vi "SDK Sample.vi"() -> ()   [LabVIEW 2015]
uses:
  sub/Mode.ctl
  sub/global.vi
panel:
  out "Depth":i8
  out "nDeviceNoList":u32[](array[numeric])
  out "MaxSize":cluster{"pWidth":u32, "pHeight":u32}={"pWidth"=2048, "pHeight"=2048}
  out "pDetectNumInfoLV":T1
  out "SetupCover2":string
  out "SetupCover1":string
  out "FLG_LiveStop":u16(ring) items=["Live", "Get", "Stop"]
  in  "Variable":bool caption="Calibrate"
  in  "Record Option":bool caption="Calibrate"
  in  "Update:":u16(ring) items=["OFF", "ON"]
  in  "Low  Light:":u16(ring) items=["OFF", "ON"]
  in  "Save Setup":bool caption="Calibrate"
  out "RetryCount":u8
  out "FLG_LiveStop":bool
  out "ColorType":enum16{"MONO", "COLOR"}(ring)
  out "Frame":i32(slide) scale=-2046.0..2045.0
  out "RecordStatus":u16(ring) items=["Record", "WaitingTRG", "Endless", "Recording"]
  out "Resolution":cluster{"pWidth":u32, "pHeight":u32}
  out "Picture":picture
  out "Mode":T2=enum."Error"
  out "Out_IP Address":T3 caption="Info_IP Address" {"Manual_IP"."IP4" format="%.03d"; "Manual_IP"."IP3" format="%.03d"; "Manual_IP"."IP2" format="%.03d"; "Manual_IP"."IP1" format="%.03d"; "Auto_IP"."IP3" format="%.03d"; "Auto_IP"."IP2" format="%.03d"; "Auto_IP"."IP1" format="%.03d"}
  out "nInterfaceCode":u32 format="%.0x"
  in  "stop":bool caption="停止"
  in  "Tab":enum32{"Camera", "Data Save", "File View"}(tab)
  in  "Record":bool caption="Calibrate"
  in  "RecStop":bool caption="Calibrate"
  in  "Setup":T4={"Frame Rate:"=0, "Shutter:"=0, "Resolution:"=4, "Trigger Mode:"=0, "Shading:"=0, "Partition:"=1, "Camera Option"=FALSE, "CameraInfo"={"Head:"=0, "Camera:"=0}} {"CameraInfo"."Camera:" items=["FASTCAM SA4 model 500K-M1"]; "CameraInfo"."Head:" items=["Head No.1"]; "Shading:" items=["Shading"]; "Shutter:" items=["1/50 sec", "1/60 sec", "1/100 sec", "1/200 sec", "1/300 sec", "1/400 sec", "1/500 sec", "1/600 sec", "1/700 sec", "1/800 sec", "1/900 sec", "1/1000 sec", "1/2000 sec", "1/3000 sec", "1/4000 sec", "1/5000 sec", "1/6000 sec", "1/7000 sec", "1/8000 sec", "1/9000 sec", "1/10000 sec", "1/12000 sec", "1/15000 sec", "1/17000 sec", "1/20000 sec", "1/25000 sec", "1/30000 sec", "1/34000 sec", "1/39000 sec", "1/50000 sec", "1/57000 sec", "1/62000 sec", "1/74000 sec", "1/82000 sec", "1/92000 sec", "1/104000 sec", "1/178000 sec", "1/333000 sec", "1/593000 sec", "1/1000000 sec"]; "Trigger Mode:" items=["START", "CENTER", "END", "MANUAL", "RANDOM", "RANDOM_RESET", "RANDOM_CENTER", "RANDOM_MANUAL", "TWOSTAGE_1/2", "TWOSTAGE_1/4", "TWOSTAGE_1/8"]; "Frame Rate:" items=["50 fps", "60 fps", "125 fps", "250 fps", "500 fps", "1000 fps", "2000 fps", "3000 fps", "3600 fps", "4500 fps", "5000 fps", "6000 fps", "6750 fps", "8000 fps", "10000 fps", "13500 fps", "20000 fps", "30000 fps", "40000 fps", "50000 fps", "60000 fps", "75000 fps", "86400 fps", "100000 fps", "150000 fps", "225000 fps", "360000 fps", "500000 fps"]; "Resolution:" items=["1024 X 1024", "1024 X 896", "1024 X 800", "1024 X 640", "1024 X 512", "896 X 896", "896 X 752", "896 X 640", "896 X 512", "768 X 768", "768 X 640", "768 X 512", "640 X 640", "512 X 512", "512 X 384", "512 X 352", "384 X 288", "320 X 240", "320 X 192", "320 X 160", "320 X 128", "256 X 256", "256 X 128", "256 X 64", "192 X 128", "128 X 128", "128 X 96", "128 X 64", "128 X 32", "128 X 16", "64 X 16"]; "Partition:" items=["Partition 1"=1, "Partition 2"=2, "Partition 3"=3, "Partition 4"=4, "Partition 5"=5, "Partition 6"=6]}
  in  "Display:":enum32{"Live", "Mem", "LiveStop"}(radio)
  in  "DataSaveInfo":T5={"DS-Format"=2, "DS-File name:"="", "DS-Save Path"=path "", "DS-Head"=0, "DS-Save"=FALSE, "Data_Slide"=0, "PLAY"=FALSE, "STOP"=FALSE, "StartFrame"=0, "EndFrame"=0, "CurrentFrame"=0, "DS-Camera:"=0} {"DS-Camera:" items=["FASTCAM SA4 model 500K-M1"]; "CurrentFrame" min=-2046 max=8871 step=1; "EndFrame" min=-2046 max=8871 step=1; "StartFrame" min=-2046 max=8871 step=1; "Data_Slide" scale=-2046.0..8871.0; "DS-Head" items=["Head No.1"]; "DS-Format" items=["BMP", "JPEG", "AVI"]}
  # "．"
  # "．"
  # "．"
  # "．"
  # "．"
  # "．"
  # "XXX"
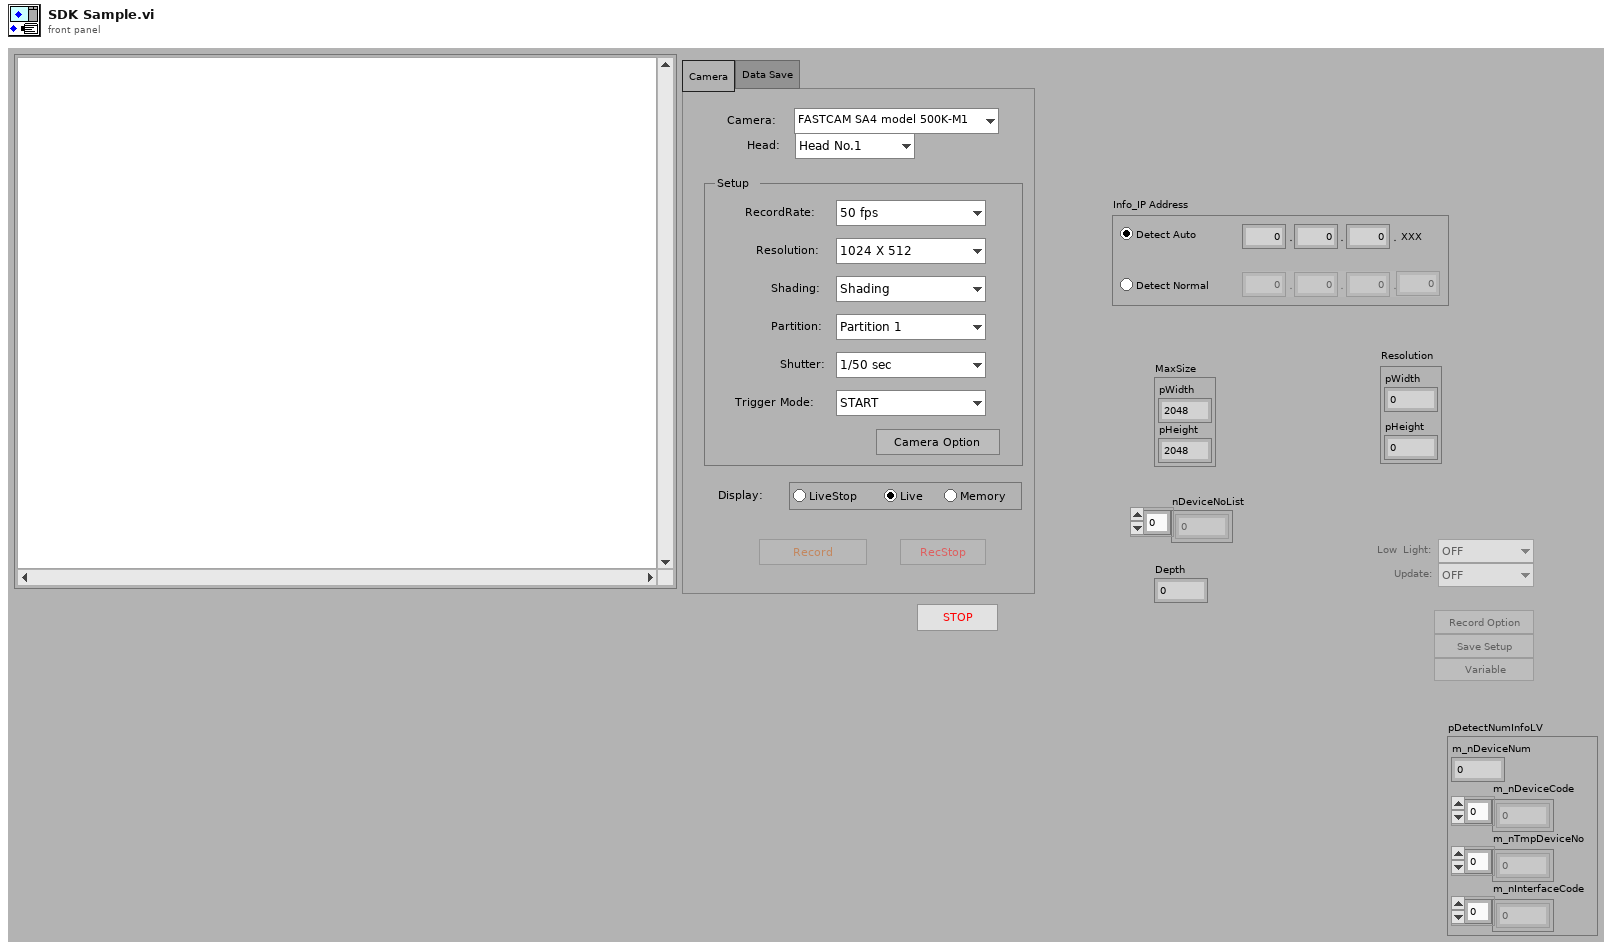
[diagram p1: front panel]
types:
  T1 = cluster{"m_nDeviceNum":u32, "m_nDeviceCode":u32[], "m_nTmpDeviceNo":u32[], "m_nInterfaceCode":u32[]}
  T2 = typedef "Mode.ctl" = enum16{"Default", "Error", "End", "Init", "DetectDevice", "Open", "Close", "GetDeviceName", "GetExistChildDeviceList", "GetColorType", "GetBitDepth.vi", "GetRecordRateList", "GetRecordRate", "SetRecordRate", "GetShutterSpeedFpsList", "GetShutterSpeedFps", "SetShutterSpeedFps", "GetResolutionList", "GetResolution", "SetResolution", "GetTriggerModeList", "GetTriggerMode", "SetTriggerMode", "GetPartitionList", "SetPartitionList", "GetCurrentPartition", "SetCurrentPartition", "GetShadingModeList", "DataSave"}
  T3 = cluster{"Detect Select BOX":enum32{"Detect Auto", "Detect Normal"}, "Auto_IP":cluster{"IP1":u8, "IP2":u8, "IP3":u8}, "Manual_IP":cluster{"IP1":u8, "IP2":u8, "IP3":u8, "IP4":u8}}
  T4 = cluster{"Frame Rate:":u16, "Shutter:":u16, "Resolution:":u16, "Trigger Mode:":u16, "Shading:":u16, "Partition:":u16, "Camera Option":bool, "CameraInfo":cluster{"Head:":u16, "Camera:":u16}}
  T5 = cluster{"DS-Format":u16, "DS-File name:":string, "DS-Save Path":path, "DS-Head":u16, "DS-Save":bool, "Data_Slide":i32, "PLAY":bool, "STOP":bool, "StartFrame":i32, "EndFrame":i32, "CurrentFrame":i32, "DS-Camera:":u16}
  T6 = enum32{"Page Enabled", "Page Disabled", "Page Disabled & Grayed"}
  T7 = cluster{"return type":u32, "pErrorCode":u32, "error ":errorcluster}
  T8 = cluster{"ReturnValue":u32, "ErrorCode":u32, "error ":errorcluster}
  T9 = cluster{"Start":i32, "End":i32, "Trigger":i32, "TwoStageLowToHigh":i32, "TwoStageHighToLow":i32, "TwoStageTiming":u32, "Event":i32[], "EventCount":u32, "RecordedFrames":u32}
  T10 = typedef "imagedata.ctl" = cluster{"image type":i32, "image depth":i32, "image":u8[], "mask":u8[], "colors":u32[], "Rectangle":cluster{"left":i16, "top":i16, "right":i16, "bottom":i16}}
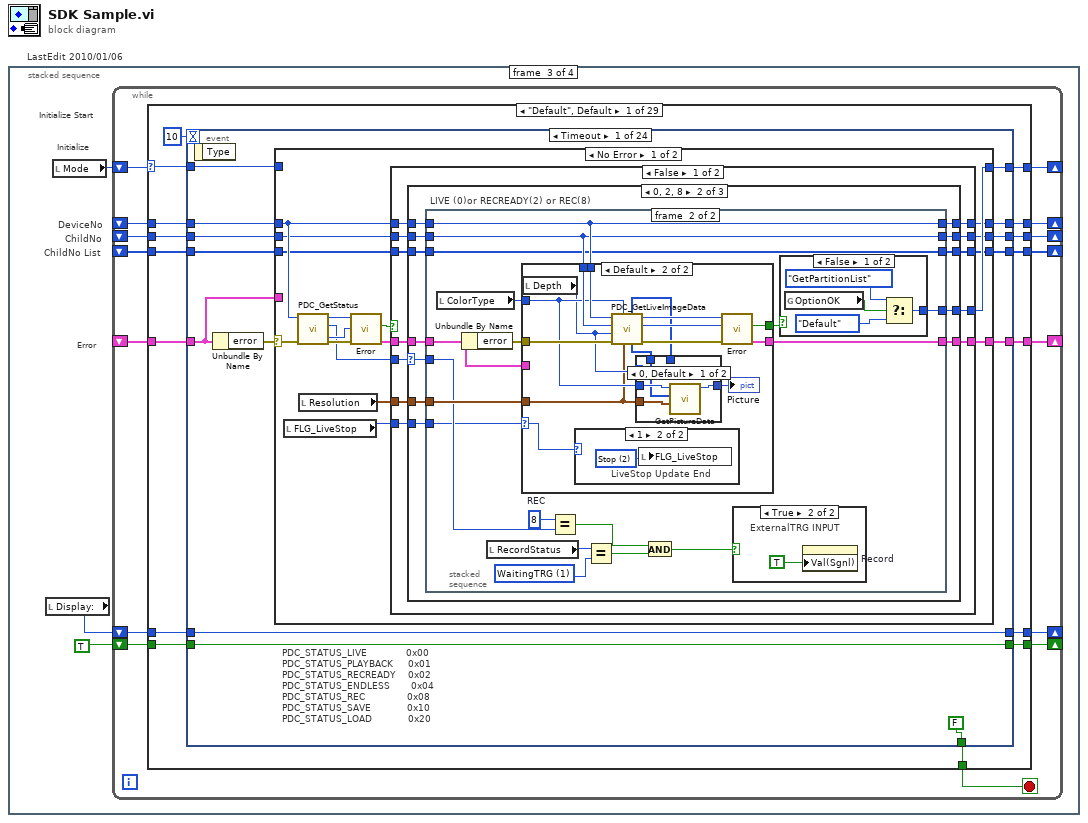
[diagram p0: block diagram]
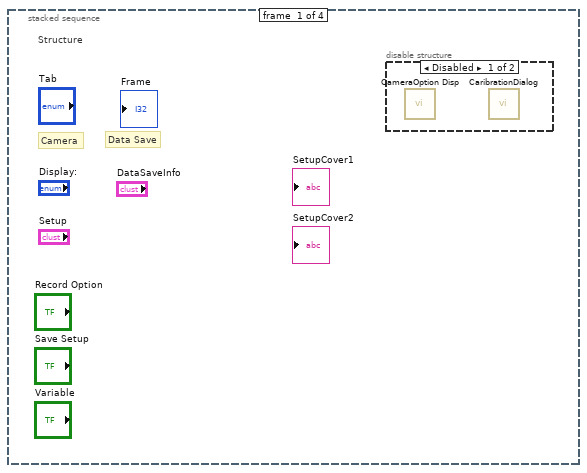
[diagram p2: hidden frame]
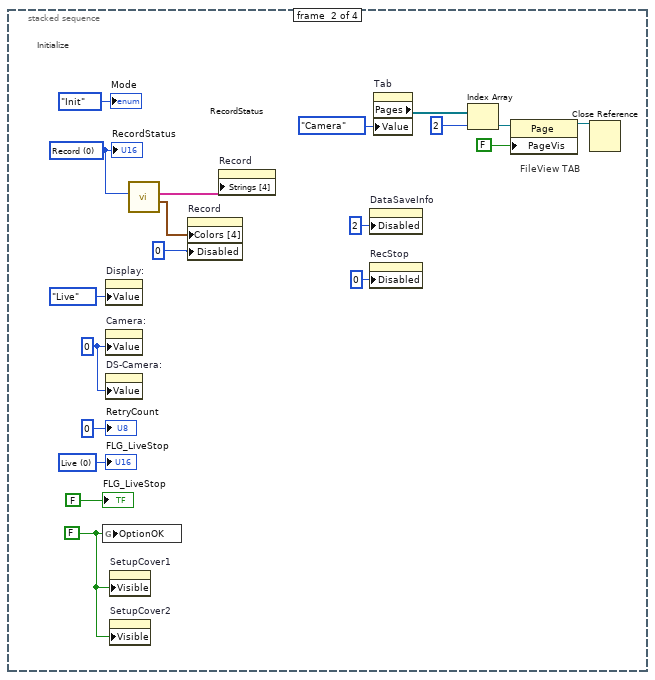
[diagram p4: hidden frame]
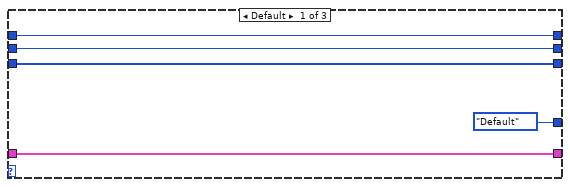
[diagram p5: hidden frame]
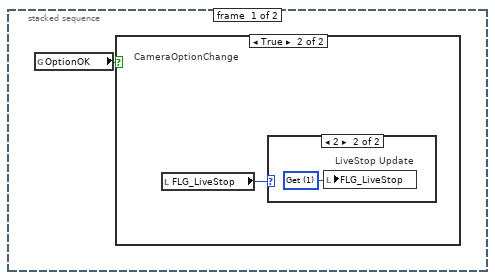
[diagram p6: hidden frame]
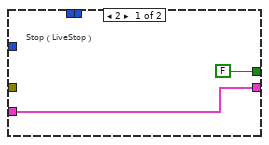
[diagram p10: hidden frame]
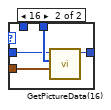
[diagram p11: hidden frame]
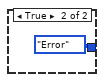
[diagram p13: hidden frame]
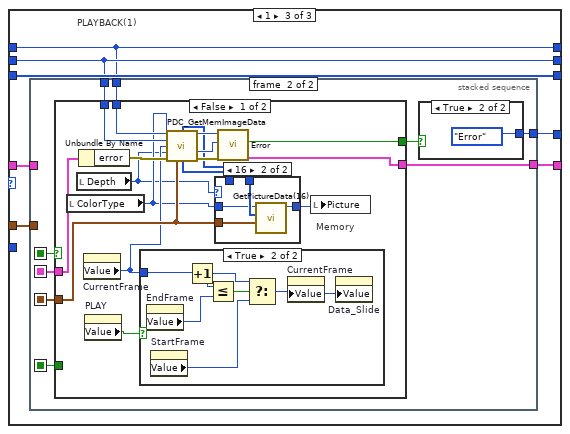
[diagram p14: hidden frame]
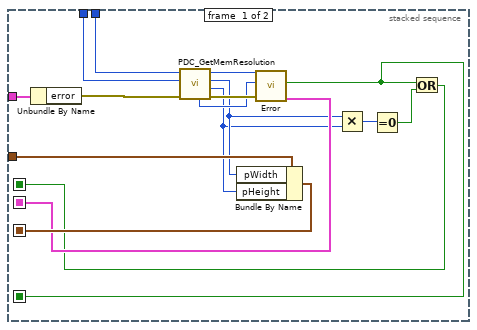
[diagram p15: hidden frame]
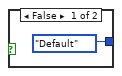
[diagram p16: hidden frame]
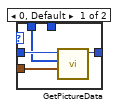
[diagram p17: hidden frame]
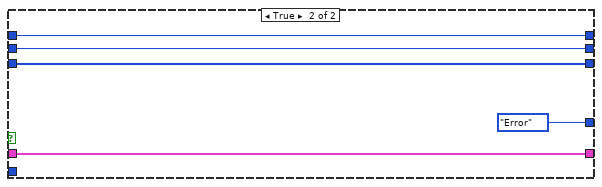
[diagram p20: hidden frame]
diagram:
  # "LastEdit 2010/01/06"
  n1 = stacked-sequence {
    frame #0 {
      # "Structure"
      # "Camera"
      # "Data Save"
      n2 = disable-structure shown="Disabled" {
        frame Disabled {
          n3 = call "CameraOption Disp.vi"() -> ()  [unwired: 12 in]
          n4 = call "CaribrationDialog.vi"() -> ()  [unwired: 1 in]
        }
        frame Enabled {
        }
      }
    }
    frame #1 {
      w2 = u16 0 ("値")
      w3 = FALSE ("OptionOK")
      w4 = u16 0 items=["Live", "Get", "Stop"] ("FLG_LiveStop")
      w19 = u16 0 items=["Record", "WaitingTRG", "Endless", "Recording"] ("RecordStatus")
      # "FileView TAB"
      # "Initialize"
      n5 = global write "global.vi" "OptionOK"(w3) -> ()
      n6 = property on="Display:" class="RadioBtnsControl (strict)"("Value"=enum32{"Live", "Mem", "LiveStop"}."Live" ("Display:")) -> ()  [unwired: 2 in, 2 out]
      n7 = property on="Camera:" class="Ring (strict)"("Value"=w2) -> ()  [unwired: 2 in, 2 out]
      n8 = property on="DS-Camera:" class="Ring (strict)"("Value"=w2) -> ()  [unwired: 2 in, 2 out]
      n9 = property on="SetupCover1" class="Str"("Visible"=w3) -> ()  [unwired: 2 in, 2 out]
      n10 = property on="SetupCover2" class="Str"("Visible"=w3) -> ()  [unwired: 2 in, 2 out]
      n11 = call "RecordStatus.vi"("RecordStatus"=w19) -> ("Color[4]"=w17:cluster{u32, u32}[], "String[4]"=w18:string[])  [unwired: 9 out]
      n12 = property on="Record" class="Bool (strict)"("Colors [4]"=w17, "Disabled"=u8 0 ("無効")) -> ()  [unwired: 2 in, 2 out]
      n13 = property on="Record" class="Bool (strict)"("Strings [4]"=w18) -> ()  [unwired: 2 in, 2 out]
      n14 = property on="DataSaveInfo" class="Clust (strict)"("Disabled"=u8 2 ("無効")) -> ()  [unwired: 2 in, 2 out]
      n15 = property on="RecStop" class="Bool (strict)"("Disabled"=u8 0 ("無効")) -> ()  [unwired: 2 in, 2 out]
      n16 = property on="Tab" class="TabCtl (strict)"("Value"=enum32{"Camera", "Data Save", "File View"}."Camera" ("Tab")) -> ("Pages"=w11:refnum<vi>[])  [unwired: 2 in, 2 out]
      n17 = Index Array(array=w11, index=2 ("指標")) -> (element=w13:refnum<vi>)
      n18 = property class="Page"(reference=w13, "PageVis"=FALSE ("ページ表示")) -> (reference out=w15:refnum<vi>)  [unwired: 1 in, 1 out]
      n19 = Close Reference(reference=w15) -> ()  [unwired: 1 in, 1 out]
      "Mode" <- Mode."Init" ("Mode")
      "RecordStatus" <- w19
      "FLG_LiveStop" <- FALSE ("FLG_LiveStop")
      "RetryCount" <- u8 0 ("RetryCount")
      "FLG_LiveStop" <- w4
    }
    frame #2 {
      # "Error"
      # "ChildNo List"
      # "Initialize"
      # "Initialize Start"
      # "ChildNo"
      # "DeviceNo"
      n20 = local read "Display:"() -> (w20:enum32{"Live", "Mem", "LiveStop"})
      n21 = local read "Mode"() -> (w22:T2)
      n22 = while {
        shift-right: [w35] -> _
        shift-left: w22 -> [w37]
        shift-right: [w33] -> _
        shift-left: _ -> [w34]
        shift-right: [w32] -> _
        shift-left: _ -> [w31]
        shift-right: [w30] -> _
        shift-left: _ -> [w29]
        shift-right: [w27] -> _
        shift-left: TRUE -> [w28]
        shift-right: [w26] -> _
        shift-left: _ -> [w25]
        shift-right: [w23] -> _
        shift-left: w20 -> [w24]
        stop <- w36 stop-if-true
        n23 = case shown="\"Default\", Default" w37 {
          selector: w37 -> [w46 _ _ _ _ _ _ _ _ _ _ _ _ _ _ _ _ _ _ _ _ _ _ _ _ _ _ _ _]
          tunnel: [w49 FALSE ("T button?") w738 FALSE ("T button?") FALSE ("T button?") FALSE ("T button?") TRUE ("T button?") FALSE ("T button?") FALSE ("T button?") FALSE ("T button?") FALSE ("T button?") FALSE ("T button?") FALSE ("T button?") FALSE ("T button?") FALSE ("T button?") FALSE ("T button?") FALSE ("T button?") FALSE ("T button?") FALSE ("T button?") FALSE ("T button?") FALSE ("T button?") FALSE ("T button?") FALSE ("T button?") FALSE ("T button?") FALSE ("T button?") FALSE ("T button?") FALSE ("T button?") FALSE ("T button?") FALSE ("T button?")] -> w36
          tunnel: w34 -> [w53 w735 w749 _ w842 w864 w899 w928 w958 w979 w997 w1020 w1048 w1073 w1096 w1126 w1150 w1179 w1215 w1248 w1268 w1291 w1309 w1343 w1365 w1387 w1399 w1426 w1475]
          tunnel: [w52 T7 {"return type"=1, "pErrorCode"=1, "error "={"status"=FALSE, "code"=0, "source"=""}} ("Error_Out") T7 {"return type"=1, "pErrorCode"=1, "error "={"status"=FALSE, "code"=0, "source"=""}} ("Error_Out") w783 w840 w863 w896 w920 w957 w977 w995 w1018 w1046 w1071 w1094 w1124 w1151 w1177 w1213 w1247 w1266 w1289 w1308 w1338 w1360 w1382 w1398 w1425 w1464] -> w33
          tunnel: [w50 Mode."Default" ("Mode") w737 w785 w843 w866 Mode."Default" ("Mode") w929 w960 w983 w1001 w1024 w1052 w1077 w1100 w1130 w1152 w1183 w1219 w1245 w1272 w1294 w1307 w1337 w1359 w1381 w1402 w1411 w1462] -> w35
          tunnel: [w47 w715 w746 w779 w834 w862 w898 w926 w955 w975 w993 w1016 w1044 w1069 w1092 w1122 w1153 w1175 w1211 w1246 w1264 w1287 w1306 w1340 w1362 w1384 w1401 w1424 w1460] -> w32
          tunnel: w31 -> [w48 w715 w746 w779 w834 _ w898 w926 w955 w975 w993 w1016 w1044 w1069 w1092 w1122 w1153 w1175 w1211 w1246 w1264 w1287 w1306 w1340 w1362 w1384 w1401 w1424 w1471]
          tunnel: [w44 w716 w747 w782 w830 w861 w897 w925 w944 w971 w990 w1008 w1034 w1061 w1084 w1113 w1139 w1170 w1199 w1231 w1261 w1284 w1305 w1339 w1361 w1383 w1400 w1423 w1461] -> w30
          tunnel: w29 -> [w45 w716 w747 w782 w830 w861 w897 w925 _ w971 w990 w1008 w1034 w1061 w1084 w1113 w1139 w1170 w1199 w1231 w1261 w1284 w1305 w1339 w1361 w1383 w1400 w1423 w1476]
          tunnel: w28 -> [w43 _ _ w781 w829 w860 w895 w924 w956 w973 w992 w1010 w1036 w1060 w1083 w1112 w1138 w1169 w1198 w1230 w1258 w1281 w1300 w1334 w1357 w1379 w1396 _ w1457]
          tunnel: [w42 FALSE FALSE w781 w829 w860 w895 w924 w956 w973 w992 w1010 w1036 w1060 w1083 w1112 w1138 w1169 w1198 w1230 w1258 w1281 w1300 w1334 w1357 w1379 w1396 FALSE ("T button?") w1457] -> w27
          tunnel: [w40 w713 w744 w780 w828 w859 w894 w922 w945 w972 w991 w1009 w1035 w1059 w1082 w1111 w1137 w1168 w1197 w1229 w1257 w1279 w1299 w1333 w1356 w1378 w1395 w1414 w1455] -> w26
          tunnel: w25 -> [w41 w713 w744 w780 w828 w859 w894 w922 _ w972 w991 w1009 w1035 w1059 w1082 w1111 w1137 w1168 w1197 w1229 w1257 w1279 w1299 w1333 w1356 w1378 w1395 w1414 w1456]
          tunnel: w24 -> [w39 w712 w743 w778 w827 w858 w893 w923 w942 w970 w989 w1007 w1033 w1058 w1081 w1110 w1136 w1167 w1196 w1228 w1256 w1278 w1298 w1332 w1355 w1377 w1394 w1413 w1454]
          tunnel: [w38 w712 w743 w778 w827 w858 w893 w923 w942 w970 w989 w1007 w1033 w1058 w1081 w1110 w1136 w1167 w1196 w1228 w1256 w1278 w1298 w1332 w1355 w1377 w1394 w1413 w1454] -> w23
          frame "Default", Default {
            n24 = event shown="[0] Timeout" {
              selector: _ -> [_ _ _ _ _ _ _ _ _ _ _ _ _ _ _ _ _ _ _ _ _ _ _ _]
              dyn-events: _ -> [_ _ _ _ _ _ _ _ _ _ _ _ _ _ _ _ _ _ _ _ _ _ _ _]
              timeout: 10 -> [_ _ _ _ _ _ _ _ _ _ _ _ _ _ _ _ _ _ _ _ _ _ _ _]
              tunnel: [FALSE ("T button?") FALSE ("T button?") FALSE ("T button?") FALSE ("T button?") FALSE ("T button?") FALSE ("T button?") FALSE ("T button?") FALSE ("T button?") FALSE ("T button?") FALSE ("T button?") FALSE ("T button?") FALSE ("T button?") FALSE ("T button?") FALSE ("T button?") FALSE ("T button?") FALSE ("T button?") FALSE ("T button?") FALSE ("T button?") FALSE ("T button?") FALSE ("T button?") FALSE ("T button?") FALSE ("T button?") FALSE ("T button?") FALSE ("T button?")] -> w49
              tunnel: w53 -> [w59 w252 w263 w279 w291 w301 w311 w320 w328 w336 w366 w398 w433 w478 w560 w585 w599 w619 w643 w654 w664 w675 w691 w700]
              tunnel: [w61 w252 w263 w279 w291 w301 w311 w320 w328 w336 w366 w395 w432 w473 w560 w585 w599 w619 w643 w654 w664 w675 w691 w700] -> w52
              tunnel: [w66 w248 Mode."GetExistChildDeviceList" ("Mode") Mode."GetColorType" ("Mode") Mode."SetRecordRate" ("Mode") Mode."SetShutterSpeedFps" ("Mode") Mode."SetResolution" ("Mode") Mode."SetTriggerMode" ("Mode") Mode."SetCurrentPartition" ("Mode") w337 w363 w393 w427 w475 w564 w588 w602 w622 w639 w651 w666 Mode."GetExistChildDeviceList" ("Mode") Mode."GetColorType" ("Mode") w696] -> w50
              tunnel: w48 -> [w65 w251 _ w280 w290 w300 w310 w319 w327 w333 w364 w390 w431 w470 w563 w587 w601 w621 w640 w652 w662 _ w690 w698]
              tunnel: [w63 w251 w260 w280 w290 w300 w310 w319 w327 w333 w364 w390 w430 w471 w563 w587 w601 w621 w640 w652 w662 w673 w690 w698] -> w47
              tunnel: w46 -> [w58 _ _ _ _ _ _ _ _ w337 w363 _ _ _ w564 w588 w602 w622 w639 w651 w666 _ _ _]
              tunnel: w45 -> [w64 w247 w265 _ w287 w297 w307 w316 w325 w332 w365 w387 w429 w469 w562 w586 w600 w620 w641 w653 w663 w677 _ w697]
              tunnel: [w62 w247 w265 w275 w287 w297 w307 w316 w325 w332 w365 w387 w428 w468 w562 w586 w600 w620 w641 w653 w663 w677 w686 w697] -> w44
              tunnel: [w57 w246 TRUE ("T button?") w277 w286 w296 w306 w315 w324 w331 w361 w385 w426 w467 w565 w582 w597 w617 w638 w648 w657 TRUE ("T button?") w689 w695] -> w42
              tunnel: w43 -> [w57 w246 _ w277 w286 w296 w306 w315 w324 w331 w361 w385 w426 w467 w565 w582 w597 w617 w638 w648 w657 _ w689 w695]
              tunnel: [w55 w245 w264 w276 w285 w295 w305 w314 w323 w330 w360 w384 w424 w464 w561 w581 w596 w616 w637 w647 w656 w676 w688 w694] -> w40
              tunnel: w41 -> [w56 w245 w264 w276 w285 w295 w305 w314 w323 w330 w360 w384 w425 w465 w561 w581 w596 w616 w637 w647 w656 w676 w688 w694]
              tunnel: w39 -> [w54 w244 w266 w269 w284 w294 w304 w313 w322 w329 w359 w383 w423 w463 w557 w580 w595 w615 w636 w646 w655 w678 w680 w693]
              tunnel: [w54 w244 w266 w269 w284 w294 w304 w313 w322 w329 w359 w383 w423 w463 w558 w580 w595 w615 w636 w646 w655 w678 w680 w693] -> w38
              event Timeout {
                # "PDC_STATUS_LIVE\t\t\t\t\t\t       0x00\nPDC_STATUS_PLAYBACK\t\t\t\t\t0x01\nPDC_STATUS_RECREADY\t\t\t\t0x02\nPDC_STATUS_ENDLESS\t\t\t\t\t  0x04\nPDC_STATUS_REC\t\t\t\t\t\t        0x08\nPDC_STATUS_SAVE\t\t\t\t\t       0x10\nPDC_STATUS_LOAD\t\t\t\t\t\t      0x20"
                n25 = event-data() -> ()  [unwired: 2 out]
                n26 = Unbundle By Name(w59) -> ("error"=w60:errorcluster)
                n27 = case shown="No Error" w60 {
                  selector: w60 -> [w71 _]
                  tunnel: [w80 w240] -> w66
                  tunnel: w65 -> [w77 w242]
                  tunnel: w64 -> [w76 w241]
                  tunnel: [w75 w242] -> w63
                  tunnel: [w74 w241] -> w62
                  tunnel: [w73 w243] -> w61
                  tunnel: w59 -> [_ w243]
                  tunnel: w58 -> [_ w240]
                  tunnel: w56 -> [w70 w239]
                  tunnel: [w69 w239] -> w55
                  frame No Error {
                    n28 = local read "FLG_LiveStop"() -> (w68:u16)
                    n29 = call "PDC_GetStatus.vi"("error in (no error)"=w71, "DeviceNo"=w77) -> ("error out"=w82:errorcluster, "Status"=w79:u32, "ReturnValue"=w84:u32, "ErrorCode"=w83:u32)  [unwired: 6 out]
                    n30 = local read "Resolution"() -> (w72:cluster{"pWidth":u32, "pHeight":u32})
                    n31 = call "Error.vi"("error in (no error)"=w82, "ErrorCode"=w83, "ReturnValue"=w84) -> ("Error_Out"=w78:T8, "Error?"=w81:bool)  [unwired: 7 out]
                    n32 = case shown="False" w81 {
                      tunnel: [w89 Mode."Error" ("Mode")] -> w80
                      tunnel: w79 -> [w96 _]
                      tunnel: w78 -> [w95 w235]
                      tunnel: w77 -> [w94 w237]
                      tunnel: w76 -> [w93 w236]
                      tunnel: [w92 w237] -> w75
                      tunnel: [w91 w236] -> w74
                      tunnel: [w90 w235] -> w73
                      tunnel: w72 -> [w88 _]
                      tunnel: w70 -> [w87 w234]
                      tunnel: [w86 w234] -> w69
                      tunnel: w68 -> [w85 _]
                      frame False {
                        n33 = case shown="0, 2, 8" w96 {
                          selector: w96 -> [_ w108 _]
                          tunnel: w95 -> [w98 w107 w172]
                          tunnel: w94 -> [w101 w113 w167]
                          tunnel: w93 -> [w100 w112 w170]
                          tunnel: [w101 w105 w167] -> w92
                          tunnel: [w100 w104 w170] -> w91
                          tunnel: [w98 w111 w169] -> w90
                          tunnel: [Mode."Default" ("Mode") w110 w168] -> w89
                          tunnel: w88 -> [_ w109 w173]
                          tunnel: [w97 w102 w171] -> w86
                          tunnel: w87 -> [w97 w103 w171]
                          tunnel: w85 -> [_ w106 _]
                          frame Default {
                          }
                          frame 0, 2, 8 {
                            # "LIVE (0)or RECREADY(2) or REC(8)"
                            n34 = stacked-sequence {
                              tunnel: w113 -> [_ w125]
                              tunnel: w112 -> [_ w124]
                              tunnel: [_ w134] -> w111
                              tunnel: [_ w132] -> w110
                              tunnel: w109 -> [_ w131]
                              tunnel: w108 -> [_ w130]
                              tunnel: w107 -> [_ w127]
                              tunnel: w106 -> [_ w126]
                              tunnel: [_ w125] -> w105
                              tunnel: [_ w124] -> w104
                              tunnel: w103 -> [_ w123]
                              tunnel: [_ w123] -> w102
                              frame #0 {
                                n35 = global read "global.vi" "OptionOK"() -> (w114:bool)
                                n36 = case shown="True" w114 {
                                frame False {
                                }
                                frame True {
                                # "CameraOptionChange"
                                n37 = local read "FLG_LiveStop"() -> (w115:u16)
                                n38 = case shown="2" w115 {
                                frame 0, Default {
                                }
                                frame 2 {
                                w116 = u16 1 items=["Live", "Get", "Stop"] ("FLG_LiveStop")
                                # "LiveStop Update"
                                n39 = local write "FLG_LiveStop"(w116) -> ()
                                }
                                }
                                }
                                }
                              }
                              frame #1 {
                                w122 = u16 1 items=["Record", "WaitingTRG", "Endless", "Recording"] ("RecordStatus")
                                w118 = u32 8  # REC
                                n40 = local read "ColorType"() -> (w128:enum16{"MONO", "COLOR"})
                                n41 = Unbundle By Name(w127) -> ("error"=w129:errorcluster)
                                n42 = local read "RecordStatus"() -> (w121:u16)
                                n43 = case shown="Default" w126 {
                                selector: w126 -> [_ w143]
                                tunnel: w125 -> [_ w152]
                                tunnel: w124 -> [_ w151]
                                tunnel: [w137 w150] -> w134
                                tunnel: [FALSE ("Error?") w149] -> w133
                                tunnel: w131 -> [_ w138]
                                tunnel: w129 -> [_ w145]
                                tunnel: w128 -> [_ w144]
                                tunnel: w127 -> [w137 _]
                                frame 2 {
                                # "Stop（LiveStop）"
                                }
                                frame Default {
                                n44 = local read "Depth"() -> (w142:i8)
                                n45 = case shown="1" w143 {
                                frame 0, Default {
                                }
                                frame 1 {
                                w161 = u16 2 items=["Live", "Get", "Stop"] ("FLG_LiveStop")
                                # "LiveStop Update End"
                                n46 = local write "FLG_LiveStop"(w161) -> ()
                                }
                                }
                                n47 = call "PDC_GetLiveImageData.vi"("Resolution"=w138, "ColorType"=w144, "error in (no error)"=w145, "BitDepth"=w142, "ChildNo"=w151, "DeviceNo"=w152) -> ("error out"=w147:errorcluster, "ErrorCode"=w141:u32, "ReturnValue"=w146:u32, "Data(8Bit)"=w140:u8[], "Data(16Bit)"=w139:u16[])  [unwired: 1 out]
                                n48 = case shown="0, Default" w142 {
                                tunnel: w138 -> [w156 w160]
                                tunnel: [w155 w159] -> w148
                                tunnel: w139 -> [_ w158]
                                tunnel: w144 -> [w154 w157]
                                tunnel: w140 -> [w153 _]
                                frame 0, Default {
                                n49 = call "GetPictureData.vi"("Resolution"=w156, "Data(8Bit)"=w153, "ColorType"=w154) -> ("new picture"=w155:picture)  [unwired: 4 out]
                                }
                                frame 16 {
                                n50 = call "GetPictureData(16).vi"("Resolution"=w160, "Data(16Bit)"=w158, "ColorType"=w157) -> ("new picture"=w159:picture)  [unwired: 4 out]
                                }
                                }
                                "Picture" <- w148
                                n51 = call "Error.vi"("error in (no error)"=w147, "ErrorCode"=w141, "ReturnValue"=w146) -> ("Error_Out"=w150:T8, "Error?"=w149:bool)  [unwired: 7 out]
                                }
                                }
                                n52 = Equal?(x=w118, y=w130) -> (x = y?=w120:bool)
                                n53 = Equal?(x=w121, y=w122) -> (x = y?=w119:bool)
                                n54 = And(x=w120, y=w119) -> (x .and. y?=w117:bool)
                                n55 = case shown="True" w117 {
                                frame False {
                                }
                                frame True {
                                # "ExternalTRG INPUT"
                                n56 = property on="Record" class="Bool (strict)"("Val(Sgnl)"=TRUE ("値 (信号)")) -> ()  [unwired: 2 in, 2 out]
                                }
                                }
                                n57 = case shown="False" w133 {
                                tunnel: [w162 Mode."Error" ("Mode")] -> w132
                                frame False {
                                n58 = global read "global.vi" "OptionOK"() -> (w165:bool)
                                n59 = Select(t=Mode."GetPartitionList" ("Mode"), s=w165, f=Mode."Default" ("Mode")) -> (s? t:f=w162:T2)
                                }
                                frame True {
                                }
                                }
                              }
                            }
                          }
                          frame 1 {
                            # "PLAYBACK(1)"
                            n60 = stacked-sequence {
                              seq-local: [w181 _] -> [_ w196]
                              seq-local: [w180 _] -> [_ w197]
                              seq-local: [w177 _] -> [_ w198]
                              seq-local: [w176 _] -> [_ w190]
                              tunnel: w173 -> [w184 _]
                              tunnel: w172 -> [w185 _]
                              tunnel: w167 -> [w183 w191]
                              tunnel: w170 -> [w182 w192]
                              tunnel: [_ w193] -> w169
                              tunnel: [_ w195] -> w168
                              frame #0 {
                                n61 = Unbundle By Name(w185) -> ("error"=w189:errorcluster)
                                n62 = call "PDC_GetMemResolution.vi"("error in (no error)"=w189, "ChildNo"=w182, "DeviceNo"=w183) -> ("error out"=w188:errorcluster, "Height"=w178:u32, "Width"=w179:u32, "ReturnValue"=w187:u32, "ErrorCode"=w186:u32)  [unwired: 4 in]
                                n63 = Bundle By Name(cluster=w184, "pWidth"=w179, "pHeight"=w178) -> (w181:cluster{"pWidth":u32, "pHeight":u32})
                                n64 = call "Error.vi"("error in (no error)"=w188, "ErrorCode"=w186, "ReturnValue"=w187) -> ("Error_Out"=w180:T8, "Error?"=w176:bool)  [unwired: 7 out]
                                n65 = Multiply(x=w179, y=w178) -> (x*y=w175:u32)
                                n66 = Equal To 0?(x=w175) -> (x = 0?=w174:bool)
                                n67 = Or(x=w176, y=w174) -> (x .or. y?=w177:bool)
                              }
                              frame #1 {
                                n68 = case shown="False" w198 {
                                tunnel: w197 -> [w206 w233]
                                tunnel: w196 -> [w207 _]
                                tunnel: [w209 w233] -> w193
                                tunnel: [w208 w232] -> w194
                                tunnel: w192 -> [w205 _]
                                tunnel: w191 -> [w204 _]
                                tunnel: w190 -> [_ w232]
                                frame False {
                                # "Memory"
                                n69 = local read "ColorType"() -> (w202:enum16{"MONO", "COLOR"})
                                n70 = local read "Depth"() -> (w201:i8)
                                n71 = Unbundle By Name(w206) -> ("error"=w213:errorcluster)
                                n72 = property on="CurrentFrame" class="DigNum (strict)"() -> ("Value"=w203:i32)  [unwired: 2 in, 2 out]
                                n73 = property on="PLAY" class="Bool (strict)"() -> ("Value"=w217:bool)  [unwired: 2 in, 2 out]
                                n74 = case shown="True" w217 {
                                tunnel: w203 -> [_ w231]
                                frame False {
                                }
                                frame True {
                                n75 = property on="EndFrame" class="DigNum (strict)"() -> ("Value"=w230:i32)  [unwired: 2 in, 2 out]
                                n76 = property on="StartFrame" class="DigNum (strict)"() -> ("Value"=w226:i32)  [unwired: 2 in, 2 out]
                                n77 = Increment(x=w231) -> (x+1=w227:i32)
                                n78 = Less Or Equal?(x=w227, y=w230) -> (x <= y?=w229:bool)
                                n79 = Select(t=w227, s=w229, f=w226) -> (s? t:f=w228:i32)
                                n80 = property on="CurrentFrame" class="DigNum (strict)"("Value"=w228) -> ()  [unwired: 2 in, 2 out]
                                n81 = property on="Data_Slide" class="Slide (strict)"("Value"=w228) -> ()  [unwired: 2 in, 2 out]
                                }
                                }
                                n82 = call "PDC_GetMemImageData.vi"("DeviceNo"=w204, "ColorType"=w202, "ChildNo"=w205, "FrameNo"=w203, "BitDepth"=w201, "error in (no error)"=w213, "Resolution"=w207) -> ("Data(16Bit)"=w211:u16[], "ReturnValue"=w215:u32, "Data(8Bit)"=w210:u8[], "ErrorCode"=w214:u32, "error out"=w216:errorcluster)  [unwired: 4 out]
                                n83 = case shown="16" w201 {
                                tunnel: w207 -> [w221 w225]
                                tunnel: [w220 w224] -> w212
                                tunnel: w211 -> [_ w223]
                                tunnel: w202 -> [w219 w222]
                                tunnel: w210 -> [w218 _]
                                frame 0, Default {
                                n84 = call "GetPictureData.vi"("Resolution"=w221, "Data(8Bit)"=w218, "ColorType"=w219) -> ("new picture"=w220:picture)  [unwired: 4 out]
                                }
                                frame 16 {
                                n85 = call "GetPictureData(16).vi"("Resolution"=w225, "Data(16Bit)"=w223, "ColorType"=w222) -> ("new picture"=w224:picture)  [unwired: 4 out]
                                }
                                }
                                n86 = call "Error.vi"("error in (no error)"=w216, "ErrorCode"=w214, "ReturnValue"=w215) -> ("Error_Out"=w209:T8, "Error?"=w208:bool)  [unwired: 7 out]
                                n87 = local write "Picture"(w212) -> ()
                                }
                                frame True {
                                }
                                }
                                n88 = case shown="True" w194 {
                                tunnel: [Mode."Default" ("Mode") Mode."Error" ("Mode")] -> w195
                                frame False {
                                }
                                frame True {
                                }
                                }
                              }
                            }
                          }
                        }
                      }
                      frame True {
                      }
                    }
                  }
                  frame Error {
                  }
                }
              }
              event "stop": Value Change {
                # "Program End"
                n89 = event-data() -> ()  [unwired: 2 out]
                n90 = Two Button Dialog(message="Exit the program" ("メッセージ"), 1:"CANCEL" ("Fボタン名(\"キャンセル\")"), 2:"OK" ("Tボタン名(\"OK\")")) -> (T button?=w249:bool)
                n91 = case shown="False" w249 {
                  tunnel: [Mode."Default" ("Mode") Mode."Close" ("Mode")] -> w248
                  frame False {
                  }
                  frame True {
                  }
                }
              }
              event "Setup.CameraInfo.Camera:": Value Change {
                n92 = event-data() -> ("NewVal"=w259:u16)  [unwired: 1 out]
                n93 = local read "nDeviceNoList"() -> (w262:u32[])
                n94 = property on="DS-Camera:" class="Ring (strict)"("Value"=w259) -> ()  [unwired: 2 in, 2 out]
                n95 = Index Array(array=w262, index=w259) -> (element=w260:u32)
              }
              event "Setup.CameraInfo.Head:": Value Change {
                w272 = FALSE ("PLAY")
                # "Push OK"
                n96 = event-data() -> ("NewVal"=w274:u16)  [unwired: 1 out]
                n97 = local read "FLG_LiveStop"() -> (w268:u16)
                n98 = property on="DS-Head" class="Ring (strict)"("Value"=w274) -> ()  [unwired: 2 in, 2 out]
                n99 = local read "DataSaveInfo"() -> (w273:T5)
                n100 = case shown="2" w268 {
                  frame 0, Default {
                  }
                  frame 2 {
                    w282 = u16 1 items=["Live", "Get", "Stop"] ("FLG_LiveStop")
                    # "LiveStop Update"
                    n101 = local write "FLG_LiveStop"(w282) -> ()
                  }
                }
                n102 = property on="PLAY" class="Bool (strict)"("Disabled"=u8 0 ("無効")) -> ()  [unwired: 2 in, 2 out]
                n103 = Index Array(array=w276, index=w274) -> (element=w275:u32)
                n104 = Bundle By Name(cluster=w273, "PLAY"=w272, "STOP"=w272) -> (w271:T5)
                n105 = local write "DataSaveInfo"(w271) -> ()
              }
              event "Setup.Frame Rate:": Value Change {
                # "Record Rate Change"
                n106 = event-data() -> ()  [unwired: 2 out]
                n107 = local read "FLG_LiveStop"() -> (w283:u16)
                n108 = case shown="2" w283 {
                  frame 0, Default {
                  }
                  frame 2 {
                    w292 = u16 1 items=["Live", "Get", "Stop"] ("FLG_LiveStop")
                    # "LiveStop Update"
                    n109 = local write "FLG_LiveStop"(w292) -> ()
                  }
                }
              }
              event "Setup.Shutter:": Value Change {
                # "Shetter Change"
                n110 = event-data() -> ()  [unwired: 2 out]
                n111 = local read "FLG_LiveStop"() -> (w293:u16)
                n112 = case shown="2" w293 {
                  frame 0, Default {
                  }
                  frame 2 {
                    w302 = u16 1 items=["Live", "Get", "Stop"] ("FLG_LiveStop")
                    # "LiveStop Update"
                    n113 = local write "FLG_LiveStop"(w302) -> ()
                  }
                }
              }
              event "Setup.Resolution:": Value Change {
                # "Resolution Change"
                n114 = event-data() -> ()  [unwired: 2 out]
                n115 = local read "FLG_LiveStop"() -> (w303:u16)
                n116 = case shown="2" w303 {
                  frame 0, Default {
                  }
                  frame 2 {
                    w312 = u16 1 items=["Live", "Get", "Stop"] ("FLG_LiveStop")
                    # "LiveStop Update"
                    n117 = local write "FLG_LiveStop"(w312) -> ()
                  }
                }
              }
              event "Setup.Trigger Mode:": Value Change {
                # "Resolution Change"
                n118 = event-data() -> ()  [unwired: 2 out]
              }
              event "Setup.Partition:": Value Change {
                # "Resolution Change"
                n119 = event-data() -> ()  [unwired: 4 out]
              }
              event "Setup.Camera Option": Value Change {
                n120 = event-data() -> ()  [unwired: 2 out]
                n121 = flat-sequence {
                  tunnel: w333 -> [w339]
                  tunnel: w332 -> [w338]
                  tunnel: [w349] -> w334
                  tunnel: w334 -> [w354]
                  frame #0 {
                    n122 = local read "Setup"() -> (w342:T4)
                    n123 = Bundle By Name(cluster=w342, "Camera Option"=FALSE) -> (w340:T4)
                    n124 = global write "global.vi" "ChildNo"(w338) -> ()
                    n125 = global write "global.vi" "DeviceNo"(w339) -> ()
                    n126 = local write "Setup"(w340) -> ()
                  }
                  frame #1 {
                    w349 = "CameraOption Disp.vi"
                    n127 = Current VI's Path() -> (path=w353:path)
                    n128 = Strip Path(path=w353) -> (stripped path=w348:path)  [unwired: 1 out]
                    n129 = Build Path(base path=w348, name or relative path="sub") -> (appended path=w346:path)
                    n130 = property on="Camera:" class="Ring (strict)"() -> ("Strings []"=w344:string[], "Value"=w345:u16)  [unwired: 2 in, 2 out]
                    n131 = Index Array(array=w344, index=w345) -> (element=w343:string)
                    n132 = Build Path(base path=w346, name or relative path=w349) -> (appended path=w352:path)
                    n133 = Open VI Reference(vi path=w352) -> (vi reference=w351:refnum<vi>)  [unwired: 1 in, 5 out]
                    n134 = property class="VI"(reference=w351, "Front Panel.Title"=w343) -> (reference out=w350:refnum<vi>)  [unwired: 1 in, 1 out]
                    n135 = Close Reference(reference=w350) -> ()  [unwired: 1 in, 1 out]
                  }
                  frame #2 {
                    # "CALL CameraOption Disp.vi"
                    n136 = call "CallDialog.vi"("vi name"=w354) -> ()  [unwired: 3 out]
                  }
                }
              }
              event "Setup.Shading:": Mouse Down {
                n137 = event-data() -> ("CtlRef"=w358:refnum<vi>)  [unwired: 1 out]
                n138 = property class="Ring (strict)"(reference=w358) -> ("Disabled"=w357:u8)  [unwired: 1 in, 2 out]
                n139 = Equal?(x=w357, y=u8 1) -> (x = y?=w355:bool)
                n140 = case shown="True" w355 {
                  tunnel: w365 -> [_ w368]
                  tunnel: w364 -> [_ w367]
                  frame False {
                    # "Not Support"
                  }
                  frame True {
                    n141 = flat-sequence {
                      tunnel: w367 -> [w372]
                      tunnel: w368 -> [w371]
                      frame #0 {
                        n142 = local read "FLG_LiveStop"() -> (w369:u16)
                        n143 = local read "Setup"() -> (w374:T4)
                        n144 = Bundle By Name(cluster=w374, "Shading:"=u16 0 ("shading:")) -> (w373:T4)
                        n145 = case shown="2" w369 {
                          frame 0, Default {
                          }
                          frame 2 {
                            w375 = u16 1 items=["Live", "Get", "Stop"] ("FLG_LiveStop")
                            # "LiveStop Update"
                            n146 = local write "FLG_LiveStop"(w375) -> ()
                          }
                        }
                        n147 = global write "global.vi" "ChildNo"(w371) -> ()
                        n148 = global write "global.vi" "DeviceNo"(w372) -> ()
                        n149 = local write "Setup"(w373) -> ()
                      }
                      frame #1 {
                        # "CALL CaribrationDialog.vi"
                        n150 = call "CallDialog.vi"("vi name"="CaribrationDialog.vi") -> ()  [unwired: 1 in, 2 out]
                      }
                    }
                  }
                }
              }
              event "Record": Value Change {
                n151 = event-data() -> ()  [unwired: 2 out]
                n152 = property on="Tab" class="TabCtl (strict)"() -> ("Pages"=w381:refnum<vi>[])  [unwired: 2 in, 2 out]
                n153 = property on="Mem" class="Bool (strict)"("Disabled"=u8 2 ("無効")) -> ()  [unwired: 2 in, 2 out]
                n154 = local read "RecordStatus"() -> (w401:u16)
                n155 = Index Array(array=w381, index=1 ("指標")) -> (element=w379:refnum<vi>)
                n156 = Unbundle By Name(w398) -> ("error"=w397:errorcluster)
                n157 = property class="Page"(reference=w379, "Page Enabled State"=T6."Page Disabled & Grayed" ("ページ使用可能状態")) -> (reference out=w377:refnum<vi>)  [unwired: 1 in, 1 out]
                n158 = case shown="3" w401 {
                  tunnel: [w410 w416 w419 w422] -> w399
                  tunnel: w397 -> [w409 w415 w417 w421]
                  tunnel: [w408 w414 w417 w421] -> w396
                  tunnel: [w407 w413 w418 w420] -> w392
                  tunnel: [w406 w412 w418 w420] -> w391
                  tunnel: w390 -> [w405 w411 _ _]
                  frame 0, Default {
                    w410 = u16 1 items=["Record", "WaitingTRG", "Endless", "Recording"] ("RecordStatus")
                    # "Recored->WaitingTRG"
                    n159 = call "PDC_SetRecReady.vi"("error in (no error)"=w409, "DeviceNo"=w405) -> ("error out"=w408:errorcluster, "ReturnValue"=w407:u32, "ErrorCode"=w406:u32)  [unwired: 7 out]
                    n160 = local write "RecordStatus"(w410) -> ()
                  }
                  frame 1 {
                    w416 = u16 3 items=["Record", "WaitingTRG", "Endless", "Recording"] ("RecordStatus")
                    # "WaitingTRG->Recording"
                    n161 = call "PDC_TriggerIn.vi"("error in (no error)"=w415, "DeviceNo"=w411) -> ("error out"=w414:errorcluster, "ReturnValue"=w413:u32, "ErrorCode"=w412:u32)  [unwired: 7 out]
                    n162 = local write "RecordStatus"(w416) -> ()
                  }
                  frame 2 {
                    w418 = u32 1 ("return type")
                    w419 = u16 3 items=["Record", "WaitingTRG", "Endless", "Recording"] ("RecordStatus")
                    # "Endless->Recording"
                    n163 = local write "RecordStatus"(w419) -> ()
                  }
                  frame 3 {
                    w420 = u32 1 ("return type")
                    w422 = u16 3 items=["Record", "WaitingTRG", "Endless", "Recording"] ("RecordStatus")
                    # "Recording"
                    n164 = local write "RecordStatus"(w422) -> ()
                  }
                }
                n165 = Close Reference(reference=w377) -> ()  [unwired: 1 in, 1 out]
                n166 = call "RecordStatus.vi"("RecordStatus"=w399) -> ("Color[4]"=w389:cluster{u32, u32}[], "String[4]"=w400:string[], "Disabled"=w388:u8)  [unwired: 8 out]
                n167 = call "Error.vi"("error in (no error)"=w396, "ErrorCode"=w391, "ReturnValue"=w392) -> ("Error_Out"=w395:T8, "Error?"=w394:bool)  [unwired: 7 out]
                n168 = property on="Record" class="Bool (strict)"("Disabled"=w388, "Strings [4]"=w400, "Colors [4]"=w389, "Value"=FALSE ("Record")) -> ()  [unwired: 2 in, 2 out]
                n169 = case shown="True" w394 {
                  tunnel: [Mode."Default" ("Mode") Mode."Error" ("Mode")] -> w393
                  frame False {
                  }
                  frame True {
                  }
                }
              }
              event "RecStop": Value Change {
                n170 = event-data() -> ()  [unwired: 2 out]
                n171 = stacked-sequence {
                  tunnel: w433 -> [_ w457]
                  tunnel: [_ w456] -> w432
                  tunnel: w431 -> [_ w455]
                  tunnel: [_ w455] -> w430
                  tunnel: w429 -> [_ w454]
                  tunnel: [_ w454] -> w428
                  tunnel: [_ w453] -> w427
                  tunnel: w425 -> [_ w446]
                  tunnel: [_ w446] -> w424
                  frame #0 {
                    w444 = u16 0 items=["Record", "WaitingTRG", "Endless", "Recording"] ("RecordStatus")
                    # "GrayScale CLEAR"
                    n172 = property on="Tab" class="TabCtl (strict)"() -> ("Pages"=w439:refnum<vi>[])  [unwired: 2 in, 2 out]
                    n173 = property on="Mem" class="Bool (strict)"("Disabled"=u8 0 ("無効")) -> ()  [unwired: 2 in, 2 out]
                    n174 = local write "RecordStatus"(w444) -> ()
                    n175 = Index Array(array=w439, index=1 ("指標")) -> (element=w437:refnum<vi>)
                    n176 = call "RecordStatus.vi"("RecordStatus"=w444) -> ("Color[4]"=w442:cluster{u32, u32}[], "String[4]"=w443:string[])  [unwired: 9 out]
                    n177 = property on="RecStop" class="Bool (strict)"("Value"=FALSE ("RecStop")) -> ()  [unwired: 2 in, 2 out]
                    n178 = property class="Page"(reference=w437, "Page Enabled State"=T6."Page Enabled" ("ページ使用可能状態")) -> (reference out=w435:refnum<vi>)  [unwired: 1 in, 1 out]
                    n179 = property on="Record" class="Bool (strict)"("Strings [4]"=w443, "Colors [4]"=w442, "Disabled"=u8 0 ("無効")) -> ()  [unwired: 2 in, 2 out]
                    n180 = Close Reference(reference=w435) -> ()  [unwired: 1 in, 1 out]
                  }
                  frame #1 {
                    w447 = u32 0  # STATUS_LIVE
                    n181 = Unbundle By Name(w457) -> ("error"=w449:errorcluster)
                    n182 = call "PDC_SetStatus.vi"("error in (no error)"=w449, "Mode"=w447, "DeviceNo"=w455) -> ("error out"=w452:errorcluster, "ReturnValue"=w451:u32, "ErrorCode"=w450:u32)  [unwired: 6 out]
                    n183 = call "Error.vi"("error in (no error)"=w452, "ErrorCode"=w450, "ReturnValue"=w451) -> ("Error_Out"=w456:T8, "Error?"=w448:bool)  [unwired: 7 out]
                    n184 = case shown="True" w448 {
                      tunnel: [Mode."Default" ("Mode") Mode."Error" ("Mode")] -> w453
                      frame False {
                      }
                      frame True {
                      }
                    }
                  }
                }
              }
              event "Display:": Value Change {
                n185 = event-data() -> ("NewVal"=w472:enum32{"Live", "Mem", "LiveStop"})  [unwired: 1 out]
                n186 = case shown="\"Mem\"" w472 {
                  tunnel: [u8 2 ("無効") u8 0 ("無効") u8 2 ("無効")] -> w483
                  tunnel: [w540 w547 w555] -> w477
                  tunnel: [u8 0 ("無効") u8 2 ("無効") u8 2 ("無効")] -> w461
                  tunnel: [u8 0 ("無効") u8 2 ("無効") u8 2 ("無効")] -> w466
                  tunnel: [w537 w544 w552] -> w462
                  tunnel: [FALSE w542 FALSE] -> w460
                  frame "Live", Default {
                    w537 = u16 0 items=["Live", "Get", "Stop"] ("FLG_LiveStop")
                    w540 = u32 0  # STATUS_LIVE
                    # "Live"
                  }
                  frame "Mem" {
                    w544 = u16 0 items=["Live", "Get", "Stop"] ("FLG_LiveStop")
                    w547 = u32 1  # STATUS_PLAYBACK
                    # "Memory"
                    n187 = local read "Tab"() -> (w543:enum32{"Camera", "Data Save", "File View"})
                    n188 = case shown="\"Data Save\"" w543 {
                      tunnel: [TRUE FALSE] -> w542
                      frame "Camera", Default {
                      }
                      frame "Data Save" {
                      }
                    }
                  }
                  frame "LiveStop" {
                    w552 = u16 1 items=["Live", "Get", "Stop"] ("FLG_LiveStop")
                    w555 = u32 0  # STATUS_LIVE
                    # "Memory"
                  }
                }
                n189 = local write "FLG_LiveStop"(w462) -> ()
                n190 = Unbundle By Name(w478) -> ("error"=w482:errorcluster)
                n191 = call "PDC_SetStatus.vi"("error in (no error)"=w482, "Mode"=w477, "DeviceNo"=w470) -> ("error out"=w481:errorcluster, "ReturnValue"=w480:u32, "ErrorCode"=w479:u32)  [unwired: 6 out]
                n192 = property on="DataSaveInfo" class="Clust (strict)"("Disabled"=w483) -> ()  [unwired: 2 in, 2 out]
                n193 = property on="Record" class="Bool (strict)"("Disabled"=w461) -> ()  [unwired: 2 in, 2 out]
                n194 = property on="RecStop" class="Bool (strict)"("Disabled"=w466) -> ()  [unwired: 2 in, 2 out]
                n195 = property on="SetupCover1" class="Str"("Visible"=w460) -> ()  [unwired: 2 in, 2 out]
                n196 = property on="SetupCover2" class="Str"("Visible"=w460) -> ()  [unwired: 2 in, 2 out]
                n197 = call "Error.vi"("error in (no error)"=w481, "ErrorCode"=w479, "ReturnValue"=w480) -> ("Error_Out"=w474:T8, "Error?"=w476:bool)  [unwired: 7 out]
                n198 = case shown="False" w476 {
                  tunnel: [w494 Mode."Error" ("Mode")] -> w475
                  tunnel: w474 -> [w492 w534]
                  tunnel: [w491 w534] -> w473
                  tunnel: w472 -> [w493 _]
                  tunnel: [w490 w533] -> w471
                  tunnel: w470 -> [w489 w533]
                  tunnel: w469 -> [w488 w532]
                  tunnel: [w487 w532] -> w468
                  tunnel: [w485 w531] -> w464
                  tunnel: w465 -> [w486 w531]
                  frame False {
                    n199 = case shown="\"Mem\"" w493 {
                      tunnel: [Mode."Default" ("Mode") w510] -> w494
                      tunnel: w492 -> [w498 w516]
                      tunnel: [w498 w511] -> w491
                      tunnel: [w497 w508] -> w490
                      tunnel: w489 -> [w497 w508]
                      tunnel: w488 -> [w496 w507]
                      tunnel: [w496 w507] -> w487
                      tunnel: [w495 w502] -> w485
                      tunnel: w486 -> [w495 w502]
                      frame Default {
                      }
                      frame "Mem" {
                        n200 = Unbundle By Name(w516) -> ("error"=w515:errorcluster)
                        n201 = call "PDC_GetMemFrameInfo.vi"("error in (no error)"=w515, "ChildNo"=w507, "DeviceNo"=w508) -> ("error out"=w514:errorcluster, "Frame"=w506:T9, "ReturnValue"=w513:u32, "ErrorCode"=w512:u32)  [unwired: 5 out]
                        n202 = Unbundle By Name(w506) -> ("Start"=w505:i32, "End"=w501:i32, "Trigger"=w500:i32)
                        n203 = To Double Precision Float(number=w501) -> (double precision float=w503:dbl)
                        n204 = To Double Precision Float(number=w505) -> (double precision float=w504:dbl)
                        n205 = call "Error.vi"("error in (no error)"=w514, "ErrorCode"=w512, "ReturnValue"=w513) -> ("Error_Out"=w511:T8, "Error?"=w509:bool)  [unwired: 7 out]
                        n206 = stacked-sequence {
                          tunnel: w505 -> [_ w520 _ _]
                          tunnel: w504 -> [w519 w522 w525 w528]
                          tunnel: w503 -> [w518 w521 w524 w527]
                          tunnel: w501 -> [_ _ _ w526]
                          tunnel: w500 -> [w517 _ w523 _]
                          frame #0 {
                            n207 = property on="Data_Slide" class="Slide (strict)"("Scale.Minimum"=w519, "Scale.Maximum"=w518, "Value"=w517) -> ()  [unwired: 2 in, 2 out]
                          }
                          frame #1 {
                            n208 = property on="StartFrame" class="DigNum (strict)"("Minimum"=w522, "Maximum"=w521, "Value"=w520) -> ()  [unwired: 2 in, 2 out]
                          }
                          frame #2 {
                            n209 = property on="CurrentFrame" class="DigNum (strict)"("Minimum"=w525, "Maximum"=w524, "Value"=w523) -> ()  [unwired: 2 in, 2 out]
                          }
                          frame #3 {
                            n210 = property on="EndFrame" class="DigNum (strict)"("Minimum"=w528, "Maximum"=w527, "Value"=w526) -> ()  [unwired: 2 in, 2 out]
                          }
                        }
                        n211 = case shown="False" w509 {
                          tunnel: [Mode."Default" ("Mode") Mode."Error" ("Mode")] -> w510
                          frame False {
                          }
                          frame True {
                          }
                        }
                      }
                    }
                  }
                  frame True {
                  }
                }
              }
              event "Tab": Value Change {
                n212 = event-data() -> ("NewVal"=w559:enum32{"Camera", "Data Save", "File View"})  [unwired: 1 out]
                n213 = case shown="\"Data Save\"" w559 {
                  tunnel: [w567 w577] -> w558
                  tunnel: w557 -> [w568 _]
                  frame "Camera", Default {
                    n214 = stacked-sequence {
                      tunnel: w568 -> [_ w573]
                      tunnel: [_ w573] -> w567
                      frame #0 {
                        w570 = FALSE ("PLAY")
                        # "Push OK"
                        n215 = local read "DataSaveInfo"() -> (w569:T5)
                        n216 = Bundle By Name(cluster=w569, "PLAY"=w570, "STOP"=w570) -> (w571:T5)
                        n217 = property on="PLAY" class="Bool (strict)"("Disabled"=u8 0 ("無効")) -> ()  [unwired: 2 in, 2 out]
                        n218 = local write "DataSaveInfo"(w571) -> ()
                      }
                      frame #1 {
                        n219 = case shown="\"Mem\"" w573 {
                          frame "Live", Default {
                            n220 = property on="Live" class="Bool (strict)"("Val(Sgnl)"=TRUE ("値 (信号)")) -> ()  [unwired: 2 in, 2 out]
                          }
                          frame "Mem" {
                            n221 = property on="Mem" class="Bool (strict)"("Val(Sgnl)"=TRUE ("値 (信号)")) -> ()  [unwired: 2 in, 2 out]
                          }
                          frame "LiveStop" {
                            n222 = property on="LiveStop" class="Bool (strict)"("Val(Sgnl)"=TRUE ("値 (信号)")) -> ()  [unwired: 2 in, 2 out]
                          }
                        }
                      }
                    }
                  }
                  frame "Data Save" {
                    n223 = stacked-sequence {
                      tunnel: [w578 _] -> w577
                      frame #0 {
                        n224 = property on="Display:" class="RadioBtnsControl (strict)"() -> ("Value"=w578:enum32{"Live", "Mem", "LiveStop"})  [unwired: 2 in, 2 out]
                      }
                      frame #1 {
                        n225 = property on="Mem" class="Bool (strict)"("Val(Sgnl)"=TRUE ("値 (信号)")) -> ()  [unwired: 2 in, 2 out]
                      }
                    }
                  }
                }
              }
              event "DataSaveInfo.Data_Slide": Value Change {
                n226 = event-data() -> ("NewVal"=w584:i32)  [unwired: 1 out]
                n227 = property on="CurrentFrame" class="DigNum (strict)"("Value"=w584) -> ()  [unwired: 2 in, 2 out]
              }
              event "DataSaveInfo.StartFrame": Value Change {
                n228 = event-data() -> ("OldVal"=w589:i32, "NewVal"=w592:i32)  [unwired: 1 out]
                n229 = property on="EndFrame" class="DigNum (strict)"() -> ("Value"=w593:i32)  [unwired: 2 in, 2 out]
                n230 = Less?(x=w592, y=w593) -> (x < y?=w591:bool)
                n231 = Greater Or Equal To 0?(x=w592) -> (x >= 0?=w594:bool)
                n232 = Compound Arithmetic op=AND(w594, w591) -> (w590:bool)
                n233 = case shown="True" w590 {
                  tunnel: w592 -> [_ w604]
                  tunnel: w589 -> [w603 _]
                  frame False {
                    n234 = property on="StartFrame" class="DigNum (strict)"("Value"=w603) -> ()  [unwired: 2 in, 2 out]
                  }
                  frame True {
                    n235 = property on="Data_Slide" class="Slide (strict)"() -> ("Value"=w605:i32)  [unwired: 2 in, 2 out]
                    n236 = flat-sequence {
                      tunnel: w604 -> [w608]
                      tunnel: w605 -> [w607]
                      frame #0 {
                        n237 = Greater?(x=w608, y=w607) -> (0:w609:bool)
                        n238 = Select(t=w608, s=w609, f=w607) -> (s? t:f=w606:i32)
                        n239 = property on="Data_Slide" class="Slide (strict)"("Scale.Minimum"=w608, "Value"=w606) -> ()  [unwired: 2 in, 2 out]
                        n240 = property on="CurrentFrame" class="DigNum (strict)"("Value"=w606) -> ()  [unwired: 2 in, 2 out]
                      }
                      frame #1 {
                        n241 = property on="STOP" class="Bool (strict)"("Val(Sgnl)"=TRUE ("値 (信号)")) -> ()  [unwired: 2 in, 2 out]
                      }
                    }
                  }
                }
              }
              event "DataSaveInfo.EndFrame": Value Change {
                n242 = event-data() -> ("OldVal"=w611:i32, "NewVal"=w614:i32)  [unwired: 1 out]
                n243 = property on="StartFrame" class="DigNum (strict)"() -> ("Value"=w613:i32)  [unwired: 2 in, 2 out]
                n244 = Greater?(x=w614, y=w613) -> (0:w612:bool)
                n245 = case shown="True" w612 {
                  tunnel: w614 -> [_ w624]
                  tunnel: w611 -> [w623 _]
                  frame False {
                    n246 = property on="EndFrame" class="DigNum (strict)"("Value"=w623) -> ()  [unwired: 2 in, 2 out]
                  }
                  frame True {
                    n247 = property on="Data_Slide" class="Slide (strict)"() -> ("Value"=w625:i32)  [unwired: 2 in, 2 out]
                    n248 = flat-sequence {
                      tunnel: w624 -> [w628]
                      tunnel: w625 -> [w627]
                      frame #0 {
                        n249 = Less?(x=w628, y=w627) -> (x < y?=w629:bool)
                        n250 = Select(t=w628, s=w629, f=w627) -> (s? t:f=w626:i32)
                        n251 = property on="Data_Slide" class="Slide (strict)"("Scale.Maximum"=w628, "Value"=w626) -> ()  [unwired: 2 in, 2 out]
                        n252 = property on="CurrentFrame" class="DigNum (strict)"("Value"=w626) -> ()  [unwired: 2 in, 2 out]
                      }
                      frame #1 {
                        n253 = property on="STOP" class="Bool (strict)"("Val(Sgnl)"=TRUE ("値 (信号)")) -> ()  [unwired: 2 in, 2 out]
                      }
                    }
                  }
                }
              }
              event "DataSaveInfo.CurrentFrame": Value Change {
                n254 = event-data() -> ("NewVal"=w633:i32)  [unwired: 1 out]
                n255 = property on="EndFrame" class="DigNum (strict)"() -> ("Value"=w635:i32)  [unwired: 2 in, 2 out]
                n256 = property on="StartFrame" class="DigNum (strict)"() -> ("Value"=w632:i32)  [unwired: 2 in, 2 out]
                n257 = In Range and Coerce(upper limit=w635, x=w633, lower limit=w632) -> (In Range?=w634:bool)  [unwired: 1 out]
                n258 = case shown="False" w634 {
                  tunnel: w633 -> [_ w645]
                  tunnel: [w644 w645] -> w631
                  tunnel: w632 -> [w644 _]
                  frame False {
                  }
                  frame True {
                  }
                }
                n259 = property on="CurrentFrame" class="DigNum (strict)"("Value"=w631) -> ()  [unwired: 2 in, 2 out]
                n260 = property on="Data_Slide" class="Slide (strict)"("Value"=w631) -> ()  [unwired: 2 in, 2 out]
              }
              event "DataSaveInfo.PLAY": Value Change {
                # "No Push"
                n261 = event-data() -> ()  [unwired: 7 out]
                n262 = property on="PLAY" class="Bool (strict)"("Disabled"=u8 1 ("無効")) -> ()  [unwired: 2 in, 2 out]
              }
              event "DataSaveInfo.STOP": Value Change {
                w660 = FALSE ("PLAY")
                # "Push OK"
                n263 = event-data() -> ()  [unwired: 2 out]
                n264 = local read "DataSaveInfo"() -> (w661:T5)
                n265 = Bundle By Name(cluster=w661, "PLAY"=w660, "STOP"=w660) -> (w659:T5)
                n266 = property on="PLAY" class="Bool (strict)"("Disabled"=u8 0 ("無効")) -> ()  [unwired: 2 in, 2 out]
                n267 = local write "DataSaveInfo"(w659) -> ()
              }
              event "DataSaveInfo.DS-Camera:": Value Change {
                w670 = FALSE ("PLAY")
                n268 = event-data() -> ("NewVal"=w668:u16)  [unwired: 1 out]
                n269 = local read "DataSaveInfo"() -> (w671:T5)
                n270 = Bundle By Name(cluster=w671, "PLAY"=w670, "STOP"=w670) -> (w669:T5)
                n271 = local write "DataSaveInfo"(w669) -> ()
                n272 = local read "nDeviceNoList"() -> (w674:u32[])
                n273 = Index Array(array=w674, index=w668) -> (element=w673:u32)
                n274 = property on="Camera:" class="Ring (strict)"("Value"=w668) -> ()  [unwired: 2 in, 2 out]
              }
              event "DataSaveInfo.DS-Head": Value Change {
                w683 = FALSE ("PLAY")
                # "Push OK"
                n275 = event-data() -> ("NewVal"=w685:u16)  [unwired: 1 out]
                n276 = property on="Head:" class="Ring (strict)"("Value"=w685) -> ()  [unwired: 2 in, 2 out]
                n277 = local read "DataSaveInfo"() -> (w684:T5)
                n278 = Index Array(array=w688, index=w685) -> (element=w686:u32)
                n279 = Bundle By Name(cluster=w684, "PLAY"=w683, "STOP"=w683) -> (w682:T5)
                n280 = property on="PLAY" class="Bool (strict)"("Disabled"=u8 0 ("無効")) -> ()  [unwired: 2 in, 2 out]
                n281 = local write "DataSaveInfo"(w682) -> ()
              }
              event "DataSaveInfo.DS-Save": Value Change {
                n282 = event-data() -> ()  [unwired: 2 out]
                n283 = flat-sequence {
                  tunnel: [w702] -> w696
                  frame #0 {
                    n284 = property on="DS-Save" class="Bool (strict)"("Value"=FALSE ("値")) -> ()  [unwired: 2 in, 2 out]
                  }
                  frame #1 {
                    n285 = local read "DataSaveInfo"() -> (w708:T5)
                    n286 = Unbundle By Name(w708) -> ("DS-Save Path"=w707:path, "DS-File name:"=w706:string)
                    n287 = Build Path(base path=w707, name or relative path=w706) -> (appended path=w705:path)
                    n288 = Not Equal?(x=w705, y=path "") -> (x != y?=w703:bool)
                    n289 = case shown="False" w703 {
                      tunnel: [Mode."Default" ("Mode") Mode."DataSave" ("Mode")] -> w702
                      frame False {
                        n290 = One Button Dialog(message="Filename Error" ("メッセージ")) -> ()  [unwired: 2 out]
                      }
                      frame True {
                      }
                    }
                  }
                }
              }
            }
          }
          frame "Error" {
            w717 = "\r\n"
            n291 = Unbundle By Name(w735) -> ("error"=w733:errorcluster, "error.source"=w730:string, "error.code"=w729:i32, "ReturnValue"=w726:u32, "ErrorCode"=w725:u32)
            n292 = Number To Decimal String(number=w729) -> (decimal integer string=w727:string)  [unwired: 1 out]
            n293 = Number To Decimal String(number=w726) -> (decimal integer string=w723:string)  [unwired: 1 out]
            n294 = Number To Decimal String(number=w725) -> (decimal integer string=w721:string)  [unwired: 1 out]
            n295 = call <vilib>:"Clear Errors.vi"("error in (no error)"=w733) -> ("error out"=w732:errorcluster)  [unwired: 1 in, 5 out]
            n296 = Concatenate Strings("<<Error !!>>", w717, w717, w717, "Source=", w730, w717, "LabError=", w727, w717, "ReturnType=", w723, w717, "ErrorCode=", w721) -> (w720:string)
            n297 = call "メッセージ表示"("error in (no error)"=w732, "Message"=w720) -> ()  [unwired: 1 in, 9 out]
          }
          frame "End" {
            n298 = local read "RetryCount"() -> (w742:u8)
            n299 = Increment(x=w742) -> (x+1=w741:u8)
            n300 = Greater Or Equal?(x=w741, y=u8 3) -> (x >= y?=w739:bool)
            n301 = local write "RetryCount"(w741) -> ()
            n302 = case shown="True" w739 {
              tunnel: w749 -> [_ w770]
              tunnel: [FALSE ("T button?") TRUE ("T button?")] -> w738
              tunnel: [Mode."Init" ("Mode") Mode."Default" ("Mode")] -> w737
              frame False {
                # "Retry"
              }
              frame True {
                w754 = "\r\n"
                n303 = Unbundle By Name(w770) -> ("error"=w769:errorcluster, "error.source"=w766:string, "error.code"=w765:i32, "ReturnValue"=w762:u32, "ErrorCode"=w761:u32)
                n304 = Number To Decimal String(number=w765) -> (decimal integer string=w763:string)  [unwired: 1 out]
                n305 = Number To Decimal String(number=w762) -> (decimal integer string=w759:string)  [unwired: 1 out]
                n306 = Number To Decimal String(number=w761) -> (decimal integer string=w757:string)  [unwired: 1 out]
                n307 = call <vilib>:"Clear Errors.vi"("error in (no error)"=w769) -> ("error out"=w768:errorcluster)  [unwired: 1 in, 5 out]
                n308 = Concatenate Strings("<<Error !!>>", w754, w754, w754, "Source=", w766, w754, "LabError=", w763, w754, "ReturnType=", w759, w754, "ErrorCode=", w757) -> (w756:string)
                n309 = call "メッセージ表示2"("error in (no error)"=w768, "Message"=w756) -> ()  [unwired: 1 in, 9 out]
              }
            }
          }
          frame "Init" {
            w773 = u32 1 ("return type")
            # "PDC_INTTYPE_G_ETHER\t\t\t0x00000002\nPDC_INTTYPE_IEEE1394\t\t\t0x00000003\nPDC_INTTYPE_PCI\t\t\t\t\t\t     0x00000100"
            n310 = call "InterfaceSelect.vi"("error in (no error)"=errorcluster {"status"=FALSE, "code"=0, "source"=""}) -> ("error out"=w774:errorcluster, "Out_IP Address"=→"Out_IP Address":T3, "nInterfaceCode"=→"nInterfaceCode":u32)  [unwired: 1 in, 7 out]
            n311 = call "Error.vi"("error in (no error)"=w774, "ErrorCode"=w773, "ReturnValue"=w773) -> ("Error_Out"=w772:T8, "Error?"=w771:bool)  [unwired: 7 out]
            n312 = case shown="False" w771 {
              tunnel: [w792 TRUE ("Error?")] -> w784
              tunnel: [w790 w804] -> w783
              tunnel: w779 -> [w788 _]
              tunnel: w772 -> [w787 w804]
              frame False {
                n313 = Unbundle By Name(w787) -> ("error"=w791:errorcluster)
                n314 = call "PDC_Init.vi"("error in (no error)"=w791) -> ("error out"=w794:errorcluster, "ErrorCode"=w789:u32, "ReturnValue"=w793:u32)  [unwired: 8 out]
                n315 = case shown="7" w789 {
                  tunnel: w794 -> [w795 w803]
                  tunnel: w793 -> [_ w802]
                  tunnel: [FALSE ("Error?") w801] -> w792
                  tunnel: [T7 {"return type"=1, "pErrorCode"=1, "error "={"status"=FALSE, "code"=0, "source"=""}} ("Error_Out") w800] -> w790
                  tunnel: w789 -> [_ w799]
                  tunnel: w788 -> [w796 _]
                  frame 7 {
                    # "既に初期化済み"
                    n316 = call "PDC_CloseDevice.vi"("error in (no error)"=w795, "DeviceNo"=w796) -> ()  [unwired: 3 in, 7 out]
                  }
                  frame Default {
                    n317 = call "Error.vi"("error in (no error)"=w803, "ErrorCode"=w799, "ReturnValue"=w802) -> ("Error_Out"=w800:T8, "Error?"=w801:bool)  [unwired: 7 out]
                  }
                }
              }
              frame True {
              }
            }
            n318 = case shown="False" w784 {
              tunnel: [Mode."DetectDevice" ("Mode") Mode."Error" ("Mode")] -> w785
              frame False {
              }
              frame True {
              }
            }
          }
          frame "DetectDevice" {
            w820 = TRUE  # NoSearch
            # "PDC_DetectDeviceLV"
            # "IP Address\nReplace"
            n319 = local read "Out_IP Address"() -> (w833:T3)
            n320 = global read "global.vi" "PDC_MAX_DEVICE"() -> (w810:i32)
            n321 = Unbundle By Name(w833) -> ("Detect Select BOX"=w832:enum32{"Detect Auto", "Detect Normal"})
            n322 = local read "nInterfaceCode"() -> (w813:u32)
            n323 = case shown="\"Detect Auto\", Default" w832 {
              tunnel: [u32 1 u32 0] -> w831
              frame "Detect Auto", Default {
              }
              frame "Detect Normal" {
              }
            }
            n324 = call "GetIPString.vi"("Out_IP Address"=w833) -> ("Net address"=w836:u32)  [unwired: 10 out]
            n325 = Initialize Array(u32 0 ("要素"), w810) -> (w838:u32[])
            n326 = Equal?(x=2, y=w813) -> (x = y?=w811:bool)
            n327 = Replace Array Subset(array=w838, new element=w836, index=0 ("指標")) -> (w835:u32[])
            n328 = Unbundle By Name(w842) -> ("error"=w841:errorcluster)
            n329 = Select(t=1, s=w811, f=w810) -> (s? t:f=w808:i32)
            n330 = call "PDC_DetectDevice.vi"("InterfaceCode"=w813, "DetectNum"=w808, "DetectParam"=w831, "error in (no error)"=w841, "DetectNo"=w835) -> ("DeviceNum"=w819:u32, "ReturnValue"=w825:u32, "DeviceCode"=w817:u32[], "TmpDeviceNo"=w816:u32[], "InterfaceCode(out)"=w815:u32[], "ErrorCode"=w824:u32, "error out"=w826:errorcluster)  [unwired: 1 in, 3 out]
            n331 = local read "pDetectNumInfoLV"() -> (w818:T1)
            n332 = Bundle By Name(cluster=w818, "m_nDeviceNum"=w819, "m_nDeviceCode"=w817, "m_nTmpDeviceNo"=w816, "m_nInterfaceCode"=w815) -> (→"pDetectNumInfoLV":T1)
            n333 = call "Error.vi"("error in (no error)"=w826, "ErrorCode"=w824, "ReturnValue"=w825) -> ("Error_Out"=w840:T8, "Error?"=w822:bool)  [unwired: 7 out]
            n334 = Equal To 0?(x=w819) -> (x = 0?=w823:bool)
            n335 = Select(t=w820, s=w823, f=w822) -> (s? t:f=w821:bool)
            n336 = case shown="False" w821 {
              tunnel: [Mode."Open" ("Mode") Mode."End" ("Mode")] -> w843
              frame False {
              }
              frame True {
                # "Retry 3times"
              }
            }
          }
          frame "Open" {
            # "<-OpenOK\n   DeviceList"
            # "DeviceSelect"
            # "ALL DeviceError->"
            # "PDC_DetectDeviceLV"
            n337 = local read "pDetectNumInfoLV"() -> (w856:T1)
            n338 = Unbundle By Name(w856) -> ("m_nDeviceNum"=w855:u32, "m_nDeviceCode"=w854:u32[], "m_nTmpDeviceNo"=w853:u32[], "m_nInterfaceCode"=w852:u32[])
            n339 = for {
              N: w855 -> [_]
              tunnel: [w871] -> w850 mode=indexing
              shift-right: [w883] -> w863
              shift-left: w864 -> [w884]
              tunnel: w854 -> [w878]
              tunnel: w853 -> [w877]
              tunnel: w852 -> [w876]
              shift-right: [w868] -> w857
              shift-left: u32[] [] ("nDeviceNoList") -> [w870]
              i -> [w875]
              n340 = Unbundle By Name(w884) -> ("error"=w880:errorcluster)
              n341 = Index Array(array=w878, index=w875) -> (element=w874:u32)
              n342 = Index Array(array=w877, index=w875) -> (element=w873:u32)
              n343 = Index Array(array=w876, index=w875) -> (element=w872:u32)
              n344 = call "PDC_OpenDevice.vi"("error in (no error)"=w880, "InterfaceCode"=w872, "TmpDeviceNo"=w873, "DeviceCode"=w874) -> ("error out"=w882:errorcluster, "DeviceNo"=w869:u32, "ErrorCode"=w879:u32, "ReturnValue"=w881:u32)  [unwired: 4 out]
              n345 = call "Error.vi"("error in (no error)"=w882, "ErrorCode"=w879, "ReturnValue"=w881) -> ("Error_Out"=w883:T8, "Error?"=w871:bool)  [unwired: 7 out]
              n346 = case shown="False" w871 {
                tunnel: w870 -> [w887 w888]
                tunnel: w869 -> [w886 _]
                tunnel: [w885 w888] -> w868
                frame False {
                  n347 = Build Array (concatenate)(w887, w886) -> (w885:u32[])
                }
                frame True {
                  # "NoDevice"
                }
              }
            }
            "nDeviceNoList" <- w857
            n348 = property on="Camera:" class="Ring (strict)"() -> ("Value"=w851:u16)  [unwired: 2 in, 2 out]
            n349 = And Array Elements(Boolean array=w850) -> (logical AND=w865:bool)
            n350 = Index Array(array=w857, index=w851) -> (element=w862:u32)
            n351 = case shown="False" w865 {
              tunnel: [Mode."GetDeviceName" ("Mode") Mode."End" ("Mode")] -> w866
              frame False {
                n352 = local write "RetryCount"(u8 0 ("RetryCount")) -> ()
              }
              frame True {
              }
            }
          }
          frame "Close" {
            n353 = local read "nDeviceNoList"() -> (w892:u32[])
            n354 = for {
              tunnel: w892 -> [w902] mode=indexing
              shift-right: [w903] -> w896
              shift-left: w899 -> [w912]
              n355 = Unbundle By Name(w912) -> ("error"=w911:errorcluster)
              n356 = call "PDC_CloseDevice.vi"("error in (no error)"=w911, "DeviceNo"=w902) -> ("error out"=w906:errorcluster, "ErrorCode"=w910:u32, "ReturnValue"=w913:u32)  [unwired: 3 in, 4 out]
              n357 = call "Error.vi"("error in (no error)"=w906, "ErrorCode"=w910, "ReturnValue"=w913) -> ("Error_Out"=w905:T8)  [unwired: 8 out]
              n358 = local read "nInterfaceCode"() -> (w908:u32)
              n359 = local read "Out_IP Address"() -> (w907:T3)
              n360 = call "Interface_RW.vi"("Mode"=enum16{"Write", "Read"}."Write", "error in (no error)"=w906, "In_IP Address"=w907, "In_InterfaceCode"=w908) -> ("error out"=w904:errorcluster)  [unwired: 7 out]
              n361 = Bundle By Name(cluster=w905, "error"=w904) -> (w903:T8)
            }
          }
          frame "GetDeviceName" {
            n362 = Unbundle By Name(w928) -> ("error"=w927:errorcluster)
            n363 = local read "nDeviceNoList"() -> (w914:u32[])
            n364 = for {
              tunnel: w914 -> [w931] mode=indexing
              tunnel: [w938] -> w921 mode=indexing
              shift-right: [w937] -> _
              shift-left: w927 -> [w939]
              tunnel: [w936] -> w920
              tunnel: [w933] -> w919 mode=indexing
              w932 = u32 0  # Device (Main set)
              n365 = call "PDC_GetDeviceName.vi"("error in (no error)"=w939, "ChildNo"=w932, "DeviceNo"=w931) -> ("error out"=w937:errorcluster, "StrName"=w938:string, "ReturnValue"=w935:u32, "ErrorCode"=w934:u32)  [unwired: 1 in, 4 out]
              n366 = call "Error.vi"("error in (no error)"=w937, "ErrorCode"=w934, "ReturnValue"=w935) -> ("Error_Out"=w936:T8, "Error?"=w933:bool)  [unwired: 7 out]
            }
            n367 = Search 1D Array(1D array=w919, element=TRUE ("要素")) -> (index of element=w917:i32)  [unwired: 1 out]
            n368 = property on="Camera:" class="Ring (strict)"("Strings []"=w921) -> ()  [unwired: 2 in, 2 out]
            n369 = property on="DS-Camera:" class="Ring (strict)"("Strings []"=w921) -> ()  [unwired: 2 in, 2 out]
            n370 = Not Equal?(x=w917, y=-1) -> (x != y?=w915:bool)
            n371 = case shown="False" w915 {
              tunnel: [Mode."GetExistChildDeviceList" ("Mode") Mode."Error" ("Mode")] -> w929
              frame False {
              }
              frame True {
              }
            }
          }
          frame "GetExistChildDeviceList" {
            w946 = u32 0 ("値")
            n372 = Unbundle By Name(w958) -> ("error"=w952:errorcluster)
            n373 = call "PDC_GetExistChildDeviceList.vi"("error in (no error)"=w952, "DeviceNo"=w955) -> ("error out"=w953:errorcluster, "List"=w945:u32[], "Size"=w951:u32, "ReturnValue"=w954:u32, "ErrorCode"=w947:u32)  [unwired: 5 out]
            n374 = for {
              N: w951 -> [_]
              tunnel: "Head No." -> [w967]
              tunnel: "%d" -> [w966]
              tunnel: [w965] -> w948 mode=indexing
              tunnel: w945 -> [w964]
              i -> [w963]
              n375 = Index Array(array=w964, index=w963) -> (element=w962:u32)
              n376 = Format Value(string ("")=w967, format string=w966, value (0)=w962) -> (output string=w965:string)
            }
            n377 = Index Array(array=w945, index=0 ("指標")) -> (element=w944:u32)
            n378 = property on="Head:" class="Ring (strict)"("Strings []"=w948, "Value"=w946) -> ()  [unwired: 2 in, 2 out]
            n379 = property on="DS-Head" class="Ring (strict)"("Strings []"=w948, "Value"=w946) -> ()  [unwired: 2 in, 2 out]
            n380 = call "Error.vi"("error in (no error)"=w953, "ErrorCode"=w947, "ReturnValue"=w954) -> ("Error_Out"=w957:T8, "Error?"=w959:bool)  [unwired: 7 out]
            n381 = case shown="False" w959 {
              tunnel: [Mode."GetColorType" ("Mode") Mode."Error" ("Mode")] -> w960
              frame False {
              }
              frame True {
              }
            }
          }
          frame "GetColorType" {
            # "PDC_COLORTYPE_MONO\t\t\t\t\t0\nPDC_COLORTYPE_COLOR\t\t\t\t1"
            n382 = Unbundle By Name(w979) -> ("error"=w978:errorcluster)
            n383 = call "PDC_GetColorType.vi"("error in (no error)"=w978, "ChildNo"=w971, "DeviceNo"=w975) -> ("error out"=w982:errorcluster, "Mode"=→"ColorType":i8, "ReturnValue"=w981:u32, "ErrorCode"=w976:u32)  [unwired: 5 out]
            n384 = call "Error.vi"("error in (no error)"=w982, "ErrorCode"=w976, "ReturnValue"=w981) -> ("Error_Out"=w977:T8, "Error?"=w980:bool)  [unwired: 7 out]
            n385 = case shown="False" w980 {
              tunnel: [Mode."GetBitDepth.vi" ("Mode") Mode."Error" ("Mode")] -> w983
              frame False {
              }
              frame True {
              }
            }
          }
          frame "GetBitDepth.vi" {
            n386 = Unbundle By Name(w997) -> ("error"=w996:errorcluster)
            n387 = call "PDC_GetBitDepth.vi"("error in (no error)"=w996, "ChildNo"=w990, "DeviceNo"=w993) -> ("error out"=w1000:errorcluster, "Depth"=w988:i8, "ReturnValue"=w999:u32, "ErrorCode"=w994:u32)  [unwired: 5 out]
            n388 = disable-structure shown="Enabled" {
              disable-tunnel: w988 -> [w1003 _]
              disable-tunnel: [w1003 i8 8 ("Depth")] -> w987
              frame Disabled {
              }
              frame Enabled {
                # "DemoProgram\n8BitONLY"
              }
            }
            "Depth" <- w987
            n389 = call "Error.vi"("error in (no error)"=w1000, "ErrorCode"=w994, "ReturnValue"=w999) -> ("Error_Out"=w995:T8, "Error?"=w998:bool)  [unwired: 7 out]
            n390 = case shown="False" w998 {
              tunnel: [Mode."GetRecordRateList" ("Mode") Mode."Error" ("Mode")] -> w1001
              frame False {
              }
              frame True {
              }
            }
          }
          frame "GetRecordRateList" {
            n391 = Unbundle By Name(w1020) -> ("error"=w1019:errorcluster)
            n392 = call "PDC_GetRecordRateList.vi"("error in (no error)"=w1019, "ChildNo"=w1008, "DeviceNo"=w1016) -> ("error out"=w1023:errorcluster, "List"=w1015:u32[], "Size"=w1011:u32, "ReturnValue"=w1022:u32, "ErrorCode"=w1017:u32)  [unwired: 4 out]
            n393 = Number To Decimal String(number=w1015) -> (decimal integer string=w1014:string[])  [unwired: 1 out]
            n394 = for {
              N: w1011 -> [_]
              tunnel: w1014 -> [w1028]
              tunnel: [w1030] -> w1013 mode=indexing
              tunnel: " fps" -> [w1029]
              i -> [w1027]
              n395 = Index Array(array=w1028, index=w1027) -> (element=w1026:string)
              n396 = Concatenate Strings(w1026, w1029) -> (w1030:string)
            }
            n397 = call "Error.vi"("error in (no error)"=w1023, "ErrorCode"=w1017, "ReturnValue"=w1022) -> ("Error_Out"=w1018:T8, "Error?"=w1021:bool)  [unwired: 7 out]
            n398 = property on="Frame Rate:" class="Ring (strict)"("Strings []"=w1013) -> ()  [unwired: 2 in, 2 out]
            n399 = case shown="False" w1021 {
              tunnel: [Mode."GetRecordRate" ("Mode") Mode."Error" ("Mode")] -> w1024
              frame False {
              }
              frame True {
              }
            }
          }
          frame "GetRecordRate" {
            n400 = Unbundle By Name(w1048) -> ("error"=w1047:errorcluster)
            n401 = call "PDC_GetRecordRate.vi"("error in (no error)"=w1047, "ChildNo"=w1034, "DeviceNo"=w1044) -> ("error out"=w1051:errorcluster, "Rate"=w1042:u32, "ReturnValue"=w1050:u32, "ErrorCode"=w1045:u32)  [unwired: 5 out]
            n402 = Number To Decimal String(number=w1042) -> (decimal integer string=w1041:string)  [unwired: 1 out]
            n403 = property on="Frame Rate:" class="Ring (strict)"() -> ("Strings []"=w1040:string[])  [unwired: 2 in, 2 out]
            n404 = Concatenate Strings(w1041, " fps") -> (w1039:string)
            n405 = call "Error.vi"("error in (no error)"=w1051, "ErrorCode"=w1045, "ReturnValue"=w1050) -> ("Error_Out"=w1046:T8, "Error?"=w1049:bool)  [unwired: 7 out]
            n406 = Search 1D Array(1D array=w1040, element=w1039) -> (index of element=w1038:i32)  [unwired: 1 out]
            n407 = case shown="-1" w1038 {
              selector: w1038 -> [w1054 _]
              tunnel: [w1054 0 ("index of element")] -> w1037
              frame Default {
              }
              frame -1 {
              }
            }
            n408 = case shown="False" w1049 {
              tunnel: [Mode."GetShutterSpeedFpsList" ("Mode") Mode."Error" ("Mode")] -> w1052
              frame False {
              }
              frame True {
              }
            }
            n409 = property on="Frame Rate:" class="Ring (strict)"("Value"=w1037) -> ()  [unwired: 2 in, 2 out]
          }
          frame "SetRecordRate" {
            n410 = property on="Frame Rate:" class="Ring (strict)"() -> ("Strings []"=w1066:string[], "Value"=w1065:u16)  [unwired: 2 in, 2 out]
            n411 = Index Array(array=w1066, index=w1065) -> (element=w1068:string)
            n412 = Match Pattern(string=w1068, regular expression=" fps") -> (before substring=w1064:string)  [unwired: 4 out]
            n413 = Unbundle By Name(w1073) -> ("error"=w1072:errorcluster)
            n414 = Decimal String To Number(string=w1064, default (0L)=u32 0 ("デフォルト (0 I32)")) -> (number=w1062:u32)  [unwired: 2 out]
            n415 = call "PDC_SetRecordRate.vi"("error in (no error)"=w1072, "Rate"=w1062, "ChildNo"=w1061, "DeviceNo"=w1069) -> ("error out"=w1076:errorcluster, "ReturnValue"=w1075:u32, "ErrorCode"=w1070:u32)  [unwired: 5 out]
            n416 = call "Error.vi"("error in (no error)"=w1076, "ErrorCode"=w1070, "ReturnValue"=w1075) -> ("Error_Out"=w1071:T8, "Error?"=w1074:bool)  [unwired: 7 out]
            n417 = case shown="False" w1074 {
              tunnel: [Mode."GetRecordRateList" ("Mode") Mode."Error" ("Mode")] -> w1077
              frame False {
              }
              frame True {
              }
            }
          }
          frame "GetShutterSpeedFpsList" {
            n418 = Unbundle By Name(w1096) -> ("error"=w1095:errorcluster)
            n419 = call "PDC_GetShutterSpeedFpsList.vi"("error in (no error)"=w1095, "ChildNo"=w1084, "DeviceNo"=w1092) -> ("error out"=w1099:errorcluster, "List"=w1089:u32[], "Size"=w1090:u32, "ReturnValue"=w1098:u32, "ErrorCode"=w1093:u32)  [unwired: 4 out]
            n420 = Number To Decimal String(number=w1089, width (-)=u32 0 ("幅（-）")) -> (decimal integer string=w1091:string[])
            n421 = for {
              N: w1090 -> [_]
              tunnel: w1091 -> [w1106]
              tunnel: [w1107] -> w1086 mode=indexing
              tunnel: "1/" -> [w1103]
              tunnel: " sec" -> [w1102]
              i -> [w1105]
              n422 = Index Array(array=w1106, index=w1105) -> (element=w1104:string)
              n423 = Concatenate Strings(w1103, w1104, w1102) -> (w1107:string)
            }
            n424 = call "Error.vi"("error in (no error)"=w1099, "ErrorCode"=w1093, "ReturnValue"=w1098) -> ("Error_Out"=w1094:T8, "Error?"=w1097:bool)  [unwired: 7 out]
            n425 = property on="Shutter:" class="Ring (strict)"("Strings []"=w1086) -> ()  [unwired: 2 in, 2 out]
            n426 = case shown="False" w1097 {
              tunnel: [Mode."GetShutterSpeedFps" ("Mode") Mode."Error" ("Mode")] -> w1100
              frame False {
              }
              frame True {
              }
            }
          }
          frame "GetShutterSpeedFps" {
            n427 = Unbundle By Name(w1126) -> ("error"=w1125:errorcluster)
            n428 = call "PDC_GetShutterSpeedFps.vi"("error in (no error)"=w1125, "ChildNo"=w1113, "DeviceNo"=w1122) -> ("error out"=w1129:errorcluster, "Fps"=w1118:u32, "ReturnValue"=w1128:u32, "ErrorCode"=w1123:u32)  [unwired: 5 out]
            n429 = Number To Decimal String(number=w1118) -> (decimal integer string=w1115:string)  [unwired: 1 out]
            n430 = property on="Shutter:" class="Ring (strict)"() -> ("Strings []"=w1117:string[])  [unwired: 2 in, 2 out]
            n431 = Concatenate Strings("1/", w1115, " sec") -> (w1120:string)
            n432 = Search 1D Array(1D array=w1117, element=w1120) -> (index of element=w1119:i32)  [unwired: 1 out]
            n433 = call "Error.vi"("error in (no error)"=w1129, "ErrorCode"=w1123, "ReturnValue"=w1128) -> ("Error_Out"=w1124:T8, "Error?"=w1127:bool)  [unwired: 7 out]
            n434 = case shown="-1" w1119 {
              selector: w1119 -> [w1132 _]
              tunnel: [w1132 0 ("index of element")] -> w1114
              frame Default {
              }
              frame -1 {
              }
            }
            n435 = property on="Shutter:" class="Ring (strict)"("Value"=w1114) -> ()  [unwired: 2 in, 2 out]
            n436 = case shown="False" w1127 {
              tunnel: [Mode."GetResolutionList" ("Mode") Mode."Error" ("Mode")] -> w1130
              frame False {
              }
              frame True {
              }
            }
          }
          frame "SetShutterSpeedFps" {
            n437 = property on="Shutter:" class="Ring (strict)"() -> ("Strings []"=w1142:string[], "Value"=w1141:u16)  [unwired: 2 in, 2 out]
            n438 = Index Array(array=w1142, index=w1141) -> (element=w1149:string)
            n439 = Match Pattern(string=w1149, regular expression=" sec") -> (before substring=w1146:string)  [unwired: 4 out]
            n440 = Match Pattern(string=w1146, regular expression="1/") -> (after substring=w1144:string)  [unwired: 4 out]
            n441 = Unbundle By Name(w1150) -> ("error"=w1155:errorcluster)
            n442 = Decimal String To Number(string=w1144, default (0L)=u32 0 ("デフォルト (0 I32)")) -> (number=w1143:u32)  [unwired: 2 out]
            n443 = call "PDC_SetShutterSpeedFps.vi"("error in (no error)"=w1155, "Fps"=w1143, "ChildNo"=w1139, "DeviceNo"=w1153) -> ("error out"=w1158:errorcluster, "ReturnValue"=w1157:u32, "ErrorCode"=w1154:u32)  [unwired: 5 out]
            n444 = call "Error.vi"("error in (no error)"=w1158, "ErrorCode"=w1154, "ReturnValue"=w1157) -> ("Error_Out"=w1151:T8, "Error?"=w1156:bool)  [unwired: 7 out]
            n445 = case shown="True" w1156 {
              tunnel: [Mode."GetRecordRateList" ("Mode") Mode."Error" ("Mode")] -> w1152
              frame False {
              }
              frame True {
              }
            }
          }
          frame "GetResolutionList" {
            n446 = Unbundle By Name(w1179) -> ("error"=w1178:errorcluster)
            n447 = call "PDC_GetResolutionList.vi"("error in (no error)"=w1178, "ChildNo"=w1170, "DeviceNo"=w1175) -> ("error out"=w1182:errorcluster, "List"=w1171:u32[], "Size"=w1174:u32, "ReturnValue"=w1181:u32, "ErrorCode"=w1176:u32)  [unwired: 4 out]
            n448 = for {
              N: w1174 -> [_]
              tunnel: " X " -> [w1191]
              tunnel: [w1190] -> w1172 mode=indexing
              tunnel: w1171 -> [w1189]
              tunnel: [w1186] -> w1166 mode=indexing
              tunnel: [w1185] -> w1165 mode=indexing
              i -> [w1188]
              n449 = Index Array(array=w1189, index=w1188) -> (element=w1187:u32)
              n450 = Split Number(x=w1187) -> (hi(x)=w1186:u16, lo(x)=w1185:u16)
              n451 = Number To Decimal String(number=w1186) -> (decimal integer string=w1193:string)  [unwired: 1 out]
              n452 = Number To Decimal String(number=w1185) -> (decimal integer string=w1192:string)  [unwired: 1 out]
              n453 = Concatenate Strings(w1193, w1191, w1192) -> (w1190:string)
            }
            n454 = call "Error.vi"("error in (no error)"=w1182, "ErrorCode"=w1176, "ReturnValue"=w1181) -> ("Error_Out"=w1177:T8, "Error?"=w1180:bool)  [unwired: 7 out]
            n455 = Array Max & Min(array=w1166) -> (max value=w1163:u16)  [unwired: 3 out]
            n456 = Array Max & Min(array=w1165) -> (max value=w1162:u16)  [unwired: 3 out]
            n457 = property on="Resolution:" class="Ring (strict)"("Strings []"=w1172) -> ()  [unwired: 2 in, 2 out]
            n458 = case shown="False" w1180 {
              tunnel: [Mode."GetResolution" ("Mode") Mode."Error" ("Mode")] -> w1183
              frame False {
              }
              frame True {
              }
            }
            n459 = local read "MaxSize"() -> (w1164:cluster{"pWidth":u32, "pHeight":u32})
            n460 = Bundle By Name(cluster=w1164, "pWidth"=w1163, "pHeight"=w1162) -> (→"MaxSize":cluster{"pWidth":u32, "pHeight":u32})
          }
          frame "GetResolution" {
            n461 = Unbundle By Name(w1215) -> ("error"=w1214:errorcluster)
            n462 = call "PDC_GetResolution.vi"("error in (no error)"=w1214, "ChildNo"=w1199, "DeviceNo"=w1211) -> ("error out"=w1218:errorcluster, "Height"=w1200:u32, "Width"=w1201:u32, "ReturnValue"=w1217:u32, "ErrorCode"=w1212:u32)  [unwired: 4 out]
            n463 = Number To Decimal String(number=w1201) -> (decimal integer string=w1208:string)  [unwired: 1 out]
            n464 = Number To Decimal String(number=w1200) -> (decimal integer string=w1209:string)  [unwired: 1 out]
            n465 = call "Error.vi"("error in (no error)"=w1218, "ErrorCode"=w1212, "ReturnValue"=w1217) -> ("Error_Out"=w1213:T8, "Error?"=w1216:bool)  [unwired: 7 out]
            n466 = property on="Resolution:" class="Ring (strict)"() -> ("Strings []"=w1206:string[])  [unwired: 2 in, 2 out]
            n467 = local read "Resolution"() -> (w1203:cluster{"pWidth":u32, "pHeight":u32})
            n468 = Concatenate Strings(w1208, " X ", w1209) -> (w1205:string)
            n469 = Bundle By Name(cluster=w1203, "pWidth"=w1201, "pHeight"=w1200) -> (→"Resolution":cluster{"pWidth":u32, "pHeight":u32})
            n470 = Search 1D Array(1D array=w1206, element=w1205) -> (index of element=w1210:i32)  [unwired: 1 in]
            n471 = case shown="-1" w1210 {
              selector: w1210 -> [w1221 _]
              tunnel: [w1221 0 ("index of element")] -> w1204
              frame Default {
              }
              frame -1 {
              }
            }
            n472 = property on="Resolution:" class="Ring (strict)"("Value"=w1204) -> ()  [unwired: 2 in, 2 out]
            n473 = case shown="False" w1216 {
              tunnel: [w1224 Mode."Error" ("Mode")] -> w1219
              tunnel: w1198 -> [w1223 _]
              frame False {
                n474 = case shown="True" w1223 {
                  tunnel: [Mode."Default" ("Mode") Mode."GetTriggerModeList" ("Mode")] -> w1224
                  frame False {
                  }
                  frame True {
                  }
                }
              }
              frame True {
              }
            }
          }
          frame "SetResolution" {
            n475 = property on="Resolution:" class="Ring (strict)"() -> ("Strings []"=w1238:string[], "Value"=w1237:u16)  [unwired: 2 in, 2 out]
            n476 = Index Array(array=w1238, index=w1237) -> (element=w1244:string)
            n477 = Match Pattern(string=w1244, regular expression=" X ") -> (before substring=w1241:string, after substring=w1239:string)  [unwired: 3 out]
            n478 = Unbundle By Name(w1248) -> ("error"=w1250:errorcluster)
            n479 = Decimal String To Number(string=w1241, default (0L)=u32 0 ("デフォルト (0 I32)")) -> (number=w1234:u32)  [unwired: 2 out]
            n480 = Decimal String To Number(string=w1239, default (0L)=u32 0 ("デフォルト (0 I32)")) -> (number=w1233:u32)  [unwired: 2 out]
            n481 = call "PDC_SetResolution.vi"("DeviceNo"=w1246, "ChildNo"=w1231, "Width"=w1234, "Height"=w1233, "error in (no error)"=w1250) -> ("ReturnValue"=w1252:u32, "ErrorCode"=w1249:u32, "error out"=w1253:errorcluster)  [unwired: 8 out]
            n482 = local read "Resolution"() -> (w1235:cluster{"pWidth":u32, "pHeight":u32})
            n483 = Bundle By Name(cluster=w1235, "pWidth"=w1234, "pHeight"=w1233) -> (w1232:cluster{"pWidth":u32, "pHeight":u32})
            n484 = local write "Resolution"(w1232) -> ()
            n485 = call "Error.vi"("error in (no error)"=w1253, "ErrorCode"=w1249, "ReturnValue"=w1252) -> ("Error_Out"=w1247:T8, "Error?"=w1251:bool)  [unwired: 7 out]
            n486 = case shown="False" w1251 {
              tunnel: [Mode."GetRecordRateList" ("Mode") Mode."Error" ("Mode")] -> w1245
              frame False {
              }
              frame True {
              }
            }
          }
          frame "GetTriggerModeList" {
            n487 = Unbundle By Name(w1268) -> ("error"=w1267:errorcluster)
            n488 = call "PDC_GetTriggerModeList.vi"("error in (no error)"=w1267, "DeviceNo"=w1264) -> ("error out"=w1271:errorcluster, "List"=w1263:u32[], "Size"=w1262:u32, "ReturnValue"=w1270:u32, "ErrorCode"=w1265:u32)  [unwired: 1 in, 4 out]
            n489 = Array Subset(array=w1263, length=w1262) -> (w1260:u32[])  [unwired: 1 in]
            n490 = for {
              tunnel: w1260 -> [w1275] mode=indexing
              tunnel: [w1274] -> w1259 mode=indexing
              n491 = call "GetTrigList.vi"("List"=w1275) -> ("Trigger mode List"=w1274:string)  [unwired: 10 out]
            }
            n492 = call "Error.vi"("error in (no error)"=w1271, "ErrorCode"=w1265, "ReturnValue"=w1270) -> ("Error_Out"=w1266:T8, "Error?"=w1269:bool)  [unwired: 7 out]
            n493 = property on="Trigger Mode:" class="Ring (strict)"("Strings []"=w1259) -> ()  [unwired: 2 in, 2 out]
            n494 = case shown="False" w1269 {
              tunnel: [Mode."GetTriggerMode" ("Mode") Mode."Error" ("Mode")] -> w1272
              frame False {
              }
              frame True {
              }
            }
          }
          frame "GetTriggerMode" {
            n495 = Unbundle By Name(w1291) -> ("error"=w1290:errorcluster)
            n496 = call "PDC_GetTriggerMode.vi"("DeviceNo"=w1287, "error in (no error)"=w1290) -> ("Mode"=w1283:u32, "ReturnValue"=w1293:u32, "ErrorCode"=w1288:u32, "error out"=w1280:errorcluster)  [unwired: 10 out]
            n497 = property on="Trigger Mode:" class="Ring (strict)"() -> ("Strings []"=w1286:string[])  [unwired: 2 in, 2 out]
            n498 = call "GetTrigList.vi"("List"=w1283) -> ("Trigger mode List"=w1282:string)  [unwired: 10 out]
            n499 = Search 1D Array(1D array=w1286, element=w1282) -> (index of element=w1285:i32)  [unwired: 1 out]
            n500 = call "Error.vi"("error in (no error)"=w1280, "ErrorCode"=w1288, "ReturnValue"=w1293) -> ("Error_Out"=w1289:T8, "Error?"=w1292:bool)  [unwired: 7 out]
            n501 = property on="Trigger Mode:" class="Ring (strict)"("Value"=w1285) -> ()  [unwired: 2 in, 2 out]
            n502 = case shown="False" w1292 {
              tunnel: [Mode."GetPartitionList" ("Mode") Mode."Error" ("Mode")] -> w1294
              frame False {
              }
              frame True {
              }
            }
          }
          frame "SetTriggerMode" {
            n503 = property on="Trigger Mode:" class="Ring (strict)"() -> ("Strings []"=w1304:string[], "Value"=w1303:u16)  [unwired: 2 in, 2 out]
            n504 = Index Array(array=w1304, index=w1303) -> (element=w1302:string)
            n505 = case shown="Default" w1302 {
              tunnel: [u32 0 ("nMode") u32 16777216 ("nMode") u32 33554432 ("nMode") u32 67108864 ("nMode") u32 50331648 ("nMode") u32 83886080 ("nMode") u32 100663296 ("nMode") u32 117440512 ("nMode") u32 134217729 ("nMode") u32 134217730 ("nMode") u32 134217731 ("nMode")] -> w1301
              frame Default {
                # "START"
              }
              frame "CENTER" {
                # "CENTER"
              }
              frame "END" {
                # "END"
              }
              frame "RANDOM" {
                # "RANDOM"
              }
              frame "MANUAL" {
                # "MANUAL"
              }
              frame "RANDOM_RESET" {
                # "RANDOM_RESET"
              }
              frame "RANDOM_CENTER" {
                # "RANDOM_CENTER"
              }
              frame "RANDOM_MANUAL" {
                # "RANDOM_MANUAL"
              }
              frame "TWOSTAGE_1/2" {
                # "RANDOM_MANUAL"
              }
              frame "TWOSTAGE_1/4" {
                # "TWOSTAGE_1/4"
              }
              frame "TWOSTAGE_1/8" {
                # "TWOSTAGE_1/8"
              }
            }
            n506 = Unbundle By Name(w1309) -> ("error"=w1311:errorcluster)
            n507 = call "PDC_SetTriggerMode.vi"("DeviceNo"=w1306, "Mode"=w1301, "error in (no error)"=w1311) -> ("ReturnValue"=w1313:u32, "ErrorCode"=w1310:u32, "error out"=w1314:errorcluster)  [unwired: 3 in, 7 out]
            n508 = call "Error.vi"("error in (no error)"=w1314, "ErrorCode"=w1310, "ReturnValue"=w1313) -> ("Error_Out"=w1308:T8, "Error?"=w1312:bool)  [unwired: 7 out]
            n509 = case shown="False" w1312 {
              tunnel: [Mode."Default" ("Mode") Mode."Error" ("Mode")] -> w1307
              frame False {
              }
              frame True {
              }
            }
          }
          frame "GetPartitionList" {
            # "1=NotSupport\n   divided partition"
            n510 = Unbundle By Name(w1343) -> ("error"=w1342:errorcluster)
            n511 = call "PDC_GetPartitionList.vi"("DeviceNo"=w1340, "ChildNo"=w1339, "error in (no error)"=w1342) -> ("ReturnValue"=w1346:u32, "Count"=w1336:u32, "ErrorCode"=w1344:u32, "error out"=w1341:errorcluster)  [unwired: 9 out]
            n512 = To Long Integer(number=w1336) -> (32bit integer=w1330:i32)
            n513 = for {
              N: w1330 -> [_]
              tunnel: "Partition " ("文字列（\"\"）") -> [w1350]
              tunnel: [w1347] -> w1329 mode=indexing
              i -> [w1352]
              n514 = Increment(x=w1352) -> (x+1=w1348:i32)
              n515 = Format Value(string ("")=w1350, format string="%d" ("形式文字列"), value (0)=w1348) -> (output string=w1349:string)
              n516 = Bundle("output string"=w1349, w1348) -> (w1347:cluster{"output string":string, i32})  [unwired: 1 out]
            }
            n517 = call "Error.vi"("error in (no error)"=w1341, "ErrorCode"=w1344, "ReturnValue"=w1346) -> ("Error_Out"=w1338:T8, "Error?"=w1345:bool)  [unwired: 7 out]
            n518 = property on="Partition:" class="Ring (strict)"("StringsAndValues[]"=w1329) -> ()  [unwired: 2 in, 2 out]
            n519 = case shown="False" w1345 {
              tunnel: [Mode."GetCurrentPartition" ("Mode") Mode."Error" ("Mode")] -> w1337
              frame False {
              }
              frame True {
              }
            }
          }
          frame "SetPartitionList" {
            n520 = Unbundle By Name(w1365) -> ("error"=w1364:errorcluster)
            n521 = call "PDC_SetPartitionList.vi"("error in (no error)"=w1364, "ChildNo"=w1361, "DeviceNo"=w1362) -> ("error out"=w1363:errorcluster, "ReturnValue"=w1368:u32, "ErrorCode"=w1366:u32)  [unwired: 2 in, 4 out]
            n522 = call "Error.vi"("error in (no error)"=w1363, "ErrorCode"=w1366, "ReturnValue"=w1368) -> ("Error_Out"=w1360:T8, "Error?"=w1367:bool)  [unwired: 7 out]
            n523 = case shown="False" w1367 {
              tunnel: [Mode."GetCurrentPartition" ("Mode") Mode."Error" ("Mode")] -> w1359
              frame False {
              }
              frame True {
              }
            }
          }
          frame "GetCurrentPartition" {
            # "1=NotSupport\n   divided partition"
            n524 = Unbundle By Name(w1387) -> ("error"=w1386:errorcluster)
            n525 = call "PDC_GetCurrentPartition.vi"("error in (no error)"=w1386, "ChildNo"=w1383, "DeviceNo"=w1384) -> ("error out"=w1385:errorcluster, "No"=w1373:u32, "ReturnValue"=w1390:u32, "ErrorCode"=w1388:u32)  [unwired: 5 out]
            n526 = property on="Partition:" class="Ring (strict)"() -> ("Strings []"=w1376:string[])  [unwired: 2 in, 2 out]
            n527 = Array Size(array=w1376) -> (size(s)=w1375:i32)
            n528 = call "Error.vi"("error in (no error)"=w1385, "ErrorCode"=w1388, "ReturnValue"=w1390) -> ("Error_Out"=w1382:T8, "Error?"=w1389:bool)  [unwired: 7 out]
            n529 = Greater Or Equal?(x=w1375, y=w1373) -> (x >= y?=w1374:bool)
            n530 = Select(t=w1373, s=w1374, f=u32 1) -> (s? t:f=w1371:u32)
            n531 = property on="Partition:" class="Ring (strict)"("Value"=w1371) -> ()  [unwired: 2 in, 2 out]
            n532 = case shown="False" w1389 {
              tunnel: [Mode."GetShadingModeList" ("Mode") Mode."Error" ("Mode")] -> w1381
              frame False {
              }
              frame True {
              }
            }
          }
          frame "SetCurrentPartition" {
            n533 = property on="Partition:" class="Ring (strict)"() -> ("Value"=w1393:u16)  [unwired: 2 in, 2 out]
            n534 = Unbundle By Name(w1399) -> ("error"=w1404:errorcluster)
            n535 = call "PDC_SetCurrentPartition.vi"("error in (no error)"=w1404, "No"=w1393, "ChildNo"=w1400, "DeviceNo"=w1401) -> ("error out"=w1407:errorcluster, "ReturnValue"=w1406:u32, "ErrorCode"=w1403:u32)  [unwired: 5 out]
            n536 = call "Error.vi"("error in (no error)"=w1407, "ErrorCode"=w1403, "ReturnValue"=w1406) -> ("Error_Out"=w1398:T8, "Error?"=w1405:bool)  [unwired: 7 out]
            n537 = case shown="False" w1405 {
              tunnel: [Mode."Default" ("Mode") Mode."Error" ("Mode")] -> w1402
              frame False {
              }
              frame True {
              }
            }
          }
          frame "GetShadingModeList" {
            w1417 = u32 21  # PDC_ERROR_NOT_SUPPORTED
            n538 = Unbundle By Name(w1426) -> ("error"=w1427:errorcluster)
            n539 = call "PDC_GetShadingModeList.vi"("error in (no error)"=w1427, "ChildNo"=w1423, "DeviceNo"=w1424) -> ("error out"=w1429:errorcluster, "List"=w1421:u32[], "Size"=w1420:u32, "ReturnValue"=w1428:u32, "ErrorCode"=w1418:u32)  [unwired: 4 out]
            n540 = Equal?(x=w1418, y=w1417) -> (x = y?=w1416:bool)
            n541 = case shown="False" w1416 {
              tunnel: w1429 -> [w1448 _]
              tunnel: w1428 -> [w1447 _]
              tunnel: [w1446 FALSE ("Error?")] -> w1410
              tunnel: [w1445 T7 {"return type"=1, "pErrorCode"=1, "error "={"status"=FALSE, "code"=0, "source"=""}} ("Error_Out")] -> w1425
              tunnel: w1421 -> [w1444 _]
              tunnel: w1420 -> [w1443 _]
              tunnel: [w1437 u8 2 ("無効")] -> w1419
              tunnel: w1418 -> [w1436 _]
              frame False {
                w1441 = u32 2  # SHADING_ON
                n542 = call "Error.vi"("error in (no error)"=w1448, "ErrorCode"=w1436, "ReturnValue"=w1447) -> ("Error_Out"=w1445:T8, "Error?"=w1446:bool)  [unwired: 7 out]
                n543 = Array Subset(array=w1444, length=w1443) -> (w1442:u32[])  [unwired: 1 in]
                n544 = Search 1D Array(1D array=w1442, element=w1441) -> (index of element=w1440:i32)  [unwired: 1 out]
                n545 = Not Equal?(x=w1440, y=-1) -> (x != y?=w1438:bool)
                n546 = case shown="False" w1438 {
                  tunnel: [u8 2 ("無効") u8 1 ("無効")] -> w1437
                  frame False {
                  }
                  frame True {
                  }
                }
              }
              frame True {
                # "NOT_SUPPORTED ->NO_ERROR"
              }
            }
            n547 = global read "global.vi" "OptionOK"() -> (w1412:bool)
            n548 = case shown="False" w1410 {
              tunnel: [w1433 Mode."Error" ("Mode")] -> w1411
              tunnel: w1412 -> [w1434 _]
              frame False {
                n549 = Select(t=Mode."GetRecordRateList" ("Mode"), s=w1434, f=Mode."Default" ("Mode")) -> (s? t:f=w1433:T2)
                n550 = global write "global.vi" "OptionOK"(FALSE ("OptionOK")) -> ()
              }
              frame True {
              }
            }
            n551 = property on="Shading:" class="Ring (strict)"("Disabled"=w1419) -> ()  [unwired: 2 in, 2 out]
          }
          frame "DataSave" {
            n552 = local read "DataSaveInfo"() -> (w1470:T5)
            n553 = Unbundle By Name(w1475) -> ("error"=w1478:errorcluster)
            n554 = Unbundle By Name(w1470) -> ("StartFrame"=w1467:i32, "EndFrame"=w1466:i32, "DS-Save Path"=w1468:path, "DS-File name:"=w1469:string, "DS-Format"=w1459:u16)
            n555 = case shown="2" w1459 {
              tunnel: [".BMP" ".JPG" ".AVI"] -> w1474
              frame 0, Default {
                # "BMP"
              }
              frame 1 {
                # "JPEG"
              }
              frame 2 {
                # "AVI(Movie)"
              }
            }
            n556 = Bundle("StartFrame"=w1467, "EndFrame"=w1466) -> (w1465:cluster{"StartFrame":i32, "EndFrame":i32})  [unwired: 1 out]
            n557 = Concatenate Strings(w1469, w1474) -> (w1473:string)
            n558 = Build Path(base path=w1468, name or relative path=w1473) -> (appended path=w1458:path)
            n559 = Path To String(path=w1458) -> (string=w1472:string)
            n560 = case shown="2" w1459 {
              tunnel: w1478 -> [w1489 w1497 w1512]
              tunnel: w1476 -> [w1482 w1500 w1504]
              tunnel: w1472 -> [w1480 _ w1509]
              tunnel: w1471 -> [w1483 w1501 w1503]
              tunnel: w1465 -> [_ _ w1507]
              tunnel: [w1487 w1495 w1506] -> w1464
              tunnel: [w1486 w1490 w1505] -> w1463
              tunnel: [w1482 w1500 w1504] -> w1461
              tunnel: [w1483 w1501 w1503] -> w1460
              tunnel: w1458 -> [_ w1494 _]
              tunnel: w1456 -> [w1479 w1493 w1502]
              tunnel: [w1479 w1493 w1502] -> w1455
              frame 0, Default {
                # "BMP"
                n561 = property on="CurrentFrame" class="DigNum (strict)"() -> ("Value"=w1481:i32)  [unwired: 2 in, 2 out]
                n562 = call "PDC_BMPFileSave.vi"("FrameNo"=w1481, "error in (no error)"=w1489, "FileName"=w1480, "ChildNo"=w1482, "DeviceNo"=w1483) -> ("error out"=w1488:errorcluster, "ReturnValue"=w1485:u32, "ErrorCode"=w1484:u32)  [unwired: 4 out]
                n563 = call "Error.vi"("error in (no error)"=w1488, "ErrorCode"=w1484, "ReturnValue"=w1485) -> ("Error_Out"=w1487:T8, "Error?"=w1486:bool)  [unwired: 7 out]
              }
              frame 1 {
                # "ErrorStatus\nCheck"
                # "JPG"
                n564 = local read "Picture"() -> (w1492:picture)
                n565 = call <vilib>:"Picture to Pixmap.vi"("picture"=w1492) -> ("image data"=w1499:T10)  [unwired: 3 in, 7 out]
                n566 = call <vilib>:"Write JPEG File.vi"("quality (80)"=75, "error in (no error)"=w1497, "image data"=w1499, "path to JPEG file"=w1494) -> ("error out"=w1491:errorcluster)  [unwired: 7 out]
                n567 = Unbundle By Name(w1491) -> ("status"=w1490:bool)
                n568 = Bundle By Name(cluster=T7 {"return type"=1, "pErrorCode"=1, "error "={"status"=FALSE, "code"=0, "source"="Write JPEG File.vi"}} ("Error_Out"), "error"=w1491) -> (w1495:T7)
              }
              frame 2 {
                w1511 = 30  # nRate
                # "AVI"
                # "CODEC Dialog"
                n569 = control-ref of="Frame"() -> (w1508:refnum<vi>)
                n570 = call "DataSave.vi"("DeviceNo"=w1503, "FileName"=w1509, "Slide Refnum"=w1508, "ChildNo"=w1504, "Rate"=w1511, "error in (no error)"=w1512, "ShowCompreddDlg"=u32 1 ("nShowCompreddDlg"), "File_Frame"=w1507) -> ("Error?"=w1505:bool, "Error_Out"=w1506:T8)  [unwired: 6 out]
              }
            }
            n571 = case shown="True" w1463 {
              tunnel: [Mode."Default" ("Mode") Mode."Error" ("Mode")] -> w1462
              frame False {
              }
              frame True {
              }
            }
          }
        }
      }
    }
    frame #3 {
      n572 = Quit LabVIEW(quit? (T)=FALSE ("終了?(T)")) -> ()
    }
  }
